vi "main.vi"() -> ()   [LabVIEW 2024]
uses:
  DataCluster.ctl
  <vilib>/userDefined/High Color/IMAQdx.ctl
  <vilib>/vision/Image Controls.llb/IMAQ Image.ctl
  DataQueue.ctl
  SensorCluster.ctl
  DataCluster_AC_PSU.ctl
  <vilib>/Platform/TimedLoop/XDataNode/timing_clust.ctl
  <vilib>/Platform/TimedLoop/XDataNode/nitl_modes.ctl
  <vilib>/Platform/TimedLoop/XDataNode/wakeup.ctl
  0b1114db-5621-4bc7-8375-4b786bff1f6f.vi
  4e5cdf46-f112-4ee0-b7be-49a859f3bfc5.vi
  2c923024-6a10-46aa-b2f6-1d0a339bce81.vi
  <extravilib>/ChannelInstances/Tag-t'DataCluster.ctl'/Read With Abort.vi
  <extravilib>/ChannelInstances/Tag-t'DataCluster.ctl'/Write With Abort.vi
  <extravilib>/ChannelInstances/Tag-t'DataCluster.ctl'/Instantiate.vi
  <extravilib>/ChannelInstances/Tag-t'DataCluster.ctl'/EndpointRead.vi
  <extravilib>/ChannelInstances/Stream-str/Instantiate.vi
  <vilib>/Platform/browser.llb/Open URL in Default Browser (string).vi
  <vilib>/Utility/file.llb/Write Delimited Spreadsheet (string).vi
  <extravilib>/ChannelInstances/Tag-t'DataCluster.ctl'/Endpoint.vi
  <vilib>/platform/TimedLoop/XDataNode/XDataNode.xnode
  <vilib>/vision/driver/NI_Vision_Acquisition_Software.lvlib
  <extravilib>/ChannelInstances/Tag-t'DataCluster.ctl'.lvlib
  <vilib>/Platform/TimedLoop/XDataNode/XDNodeRunTimeDep.lvlib
  <resource>/objmgr/imaqdx.rc
panel:
  out "Galium Control":string="Galium Control" caption="Version"
  in  "Save Snapshot":bool
  out "Overload":bool caption="System Overloaded!"
  out "error out 3":errorcluster
  out "Auto Tune PID gains":T1
  out "TuneComplete":bool caption="Done"
  in  "AutoTune":bool
  out "error out 2":errorcluster
  out "error out":errorcluster
  out "T_Log":string="00:30:00" caption="Sample Duration"
  out "version":string="version 0.0.0.1" caption="Version"
  in  "Start":bool
  out "Title":string="BioSIM" caption="Version"
  out "cDAQ_Time":u32(graph) caption="DAQ - Process Time"
  out "DP_Overhead":i64(graph)=499 caption="Data Acquisition - Overhead"
  in  "DataCluster":T2={"Core"={"Current VI Reference"=refnum, "Close Panel on Exit?"=FALSE, "Exit"=FALSE, "Initialized?"=FALSE}, "Connections"={"cDAQ DO"={"Task"="", "Connected"=FALSE, "Active"=FALSE, "ID"=""}, "cDAQ AO"={"Task"="", "Connected"=FALSE, "Active"=FALSE, "ID"=""}, "cDAQ AI"={"Task"="", "Connected"=FALSE, "Active"=FALSE, "ID"=""}, "Camera"={"Session"="", "Connected"=FALSE, "Active"=FALSE, "Placeholder"=refnum}, "Humidity"={"Port"="", "Connected"=FALSE, "Active"=FALSE}}, "Data Acquisition"={"Setup"={"Label"="", "Operator"="", "Notes"="", "CircTemp"=1.0, "FlowRate"=1.0}, "Camera"={"Image"=refnum, "Save Image"=refnum, "Image Frequency"=20, "Rectangle"={"Left"=0, "Top"=0, "Right"=0, "Bottom"=0, "Rotation"=0.0}, "Calibration"={"Top Left"={"X"=0.0, "Y"=0.0}, "Top Right"={"X"=0.0, "Y"=0.0}, "Bottom Left"={"X"=0.0, "Y"=0.0}, "Bottom Right"={"X"=0.0, "Y"=0.0}, "Fixpoint"={"X"=0.0, "Y"=0.0}, "Scan Area"=0.0, "Fixpoint Area"=0.0, "Well Pixels"=[], "Valid"=FALSE}, "FocusPos"=0, "Display Mapping"=10}, "Thermistor"={"Sample Size"=1, "Calibration"={"B0.100"=[], "R25"=[], "c"=[], "State"=[], "V_S"=5.0, "R_S"=100.0}, "Timing Mode"=14713}, "Partition"={"Data"=[], "Cell Label"="", "Cell Color"=0, "Height"=10, "Width"=16, "Grid"=[]}, "Queue"={"Queue"=refnum, "Size"=1}, "Sample Rate"=20, "Active"=FALSE, "Ready"=FALSE, "Graph Mode"=0, "Gradient Buffer"=2}, "Control"={"Sample Rate"=1, "LogStart ms"=0, "AC PSU"={"Voltage"=0.0, "Frequency"=0.0, "State"={"15+16 - Waveform"=0, "17 - Freq Control EN"=FALSE, "18 - Voltage Output"=FALSE, "19 - Output Mode"=0, "20 - Mode Control EN"=FALSE, "21 - AC Control EN"=FALSE, "24 - DC Control EN"=FALSE, "25 - DC Polarity Bias"=FALSE}}, "DC PSU"={"Voltage"=0.0, "Active"=FALSE, "Pulse Size"=0.0, "Pulse Duration"=0.0, "Voltage Set"=0.0}, "Computer Vision"={"Target Pos"=0.0, "Current Pos"=0.0, "Processing"=refnum, "Range"={"Lower value"=128.0, "Upper value"=255.0}, "MinArea"=2, "16-bit Conversion Method"=10, "Display Image"=10, "Binary"=refnum, "Gain"=0.0, "Exposure time"=0.0}, "PID"={"AutoPID"=FALSE, "Gains"={"proportional gain (Kc)"=1.0, "integral time (Ti, min)"=0.01, "derivative time (Td, min)"=0.0}, "autotuning parameters"={"controller type"=1, "relay cycles"=3, "relay amplitude"=1.0, "control specification"=2, "PV noise level"=0.1}, "Show Controls"=FALSE}}, "Manual Temp Control"={"TargetTemp"=1.0, "Mode"=0, "Active"=FALSE}} {"Manual Temp Control"."Mode" items=["Cool", "Heat"]; "Manual Temp Control"."TargetTemp" min=-40.0 max=40.0 step=0.5 format="%#_g °C"; "Control"."PID"."autotuning parameters"."PV noise level" format="%.2f"; "Control"."PID"."autotuning parameters"."control specification" items=["normal", "fast", "slow"]; "Control"."PID"."autotuning parameters"."relay amplitude" format="%.2f"; "Control"."PID"."autotuning parameters"."controller type" items=["PID", "PI", "P"]; "Control"."PID"."Gains"."derivative time (Td, min)" format="%.3f"; "Control"."PID"."Gains"."integral time (Ti, min)" format="%.3f"; "Control"."PID"."Gains"."proportional gain (Kc)" format="%.3f"; "Control"."Computer Vision"."Display Image" items=["Default", "Computer Vision"]; "Control"."Computer Vision"."16-bit Conversion Method" items=["Default"=10, "Most Significant Bits"=11, "Full Dynamic"=12, "Downshift"=13, "Given Range"=14, "90% Dynamic"=15, "Given Percent Range"=16]; "Control"."Computer Vision"."Range"."Upper value" format="%.2f"; "Control"."Computer Vision"."Range"."Lower value" format="%.2f"; "Control"."AC PSU"."State"."19 - Output Mode" items=["Constant Voltage", "Constant Current"]; "Control"."AC PSU"."State"."15+16 - Waveform" items=["Sine", "Square", "Triangle"]; "Control"."Sample Rate" min=1 max=20 step=1 format="%.0f Samples/sec"; "Data Acquisition"."Gradient Buffer" min=2 max=30 step=1; "Data Acquisition"."Graph Mode" items=["Thermistor Temperature", "Camera Temperature"]; "Data Acquisition"."Thermistor"."Timing Mode" items=["Automatic"=16097, "High Resolution"=10195, "High Speed"=14712, "Best 50 Hz Rejection"=14713, "Best 60 Hz Rejection"=14714, "Custom"=10137]; "Data Acquisition"."Thermistor"."Calibration"."R_S" min=0.1 max=1000.0 format="%#_g kOhm"; "Data Acquisition"."Thermistor"."Calibration"."V_S" min=5.0 max=48.0 format="%#_g V"; "Data Acquisition"."Thermistor"."Calibration"."R25" min=0.1 max=1000.0 format="%#_g kOhm"; "Data Acquisition"."Thermistor"."Calibration"."B0.100" min=100.0 max=10000.0 format="%#_g K"; "Data Acquisition"."Thermistor"."Sample Size" min=1 max=200; "Data Acquisition"."Sample Rate" min=20 max=240 format="%.0f samples/min"; "Data Acquisition"."Queue"."Size" min=1 max=200; "Data Acquisition"."Camera"."Display Mapping" items=["Default"=10, "Most Significant Bits"=11, "Full Dynamic"=12, "Downshift"=13, "Given Range"=14, "90% Dynamic"=15, "Given Percent Range"=16]; "Data Acquisition"."Camera"."Calibration"."Fixpoint"."Y" format="%.2f"; "Data Acquisition"."Camera"."Calibration"."Fixpoint"."X" format="%.2f"; "Data Acquisition"."Camera"."Calibration"."Top Left"."Y" format="%.2f"; "Data Acquisition"."Camera"."Calibration"."Top Left"."X" format="%.2f"; "Data Acquisition"."Camera"."Calibration"."Top Right"."Y" format="%.2f"; "Data Acquisition"."Camera"."Calibration"."Top Right"."X" format="%.2f"; "Data Acquisition"."Camera"."Calibration"."Bottom Left"."Y" format="%.2f"; "Data Acquisition"."Camera"."Calibration"."Bottom Left"."X" format="%.2f"; "Data Acquisition"."Camera"."Calibration"."Bottom Right"."Y" format="%.2f"; "Data Acquisition"."Camera"."Calibration"."Bottom Right"."X" format="%.2f"; "Data Acquisition"."Camera"."Rectangle"."Rotation" min=-90.0 max=90.0 step=1.0 format="%.2f"; "Data Acquisition"."Camera"."Rectangle"."Left" scale=0.0..1024.0; "Data Acquisition"."Camera"."Rectangle"."Right" scale=0.0..1024.0; "Data Acquisition"."Camera"."Image Frequency" min=1 max=60 step=1; "Data Acquisition"."Setup"."FlowRate" min=0.0 max=500.0 format="%#_g L/min"; "Data Acquisition"."Setup"."CircTemp" min=-40.0 max=40.0 step=0.5 format="%#_g °C"}
  in  "Help":bool
  out "DC Volt":dbl[unit](graph)
  out "Temps":dbl[unit](graph)
  out "Processing Feed":T4(plugin-control)
  out "Camera Feed":T4(plugin-control)
  out "Air Temp.":dbl format="%#_g °C"
  out "Dewpoint":dbl format="%#_g °C"
  out "Position":dbl caption="Average Position" format="%#.6f"
  out "Temp":dbl[unit]=273.15 caption="Temperature" format="%#.6f"
  out "Humidity Status":string
  out "Temp Status":string
  out "Humidity":dbl format="%#.6f %%"
  in  "Pulse":bool
  out "DC_Status":string
  in  "DC_Voltage_Slide":u32(slide) scale=0.0..100.0
  in  "DC_Voltage":dbl[unit] caption="DC Voltage" min=0.0 max=1500.0 format="%#.0f"
  out "AC_Status":string
  in  "AC_Voltage_Slide":u32(slide) scale=0.0..100.0
  in  "AC_Freq":dbl[unit]=100.0 caption="AC Frequency" min=100.0 max=10000.0 format="%#.0f"
  in  "AC_Voltage":dbl[unit] caption="AC Voltage" min=0.0 max=10000.0
  in  "AC_Freq_Slide":u32(slide) scale=0.0..100.0
  out "StatusString":string="Closing System"
  # "Bioaerosol Simulation Chamber"
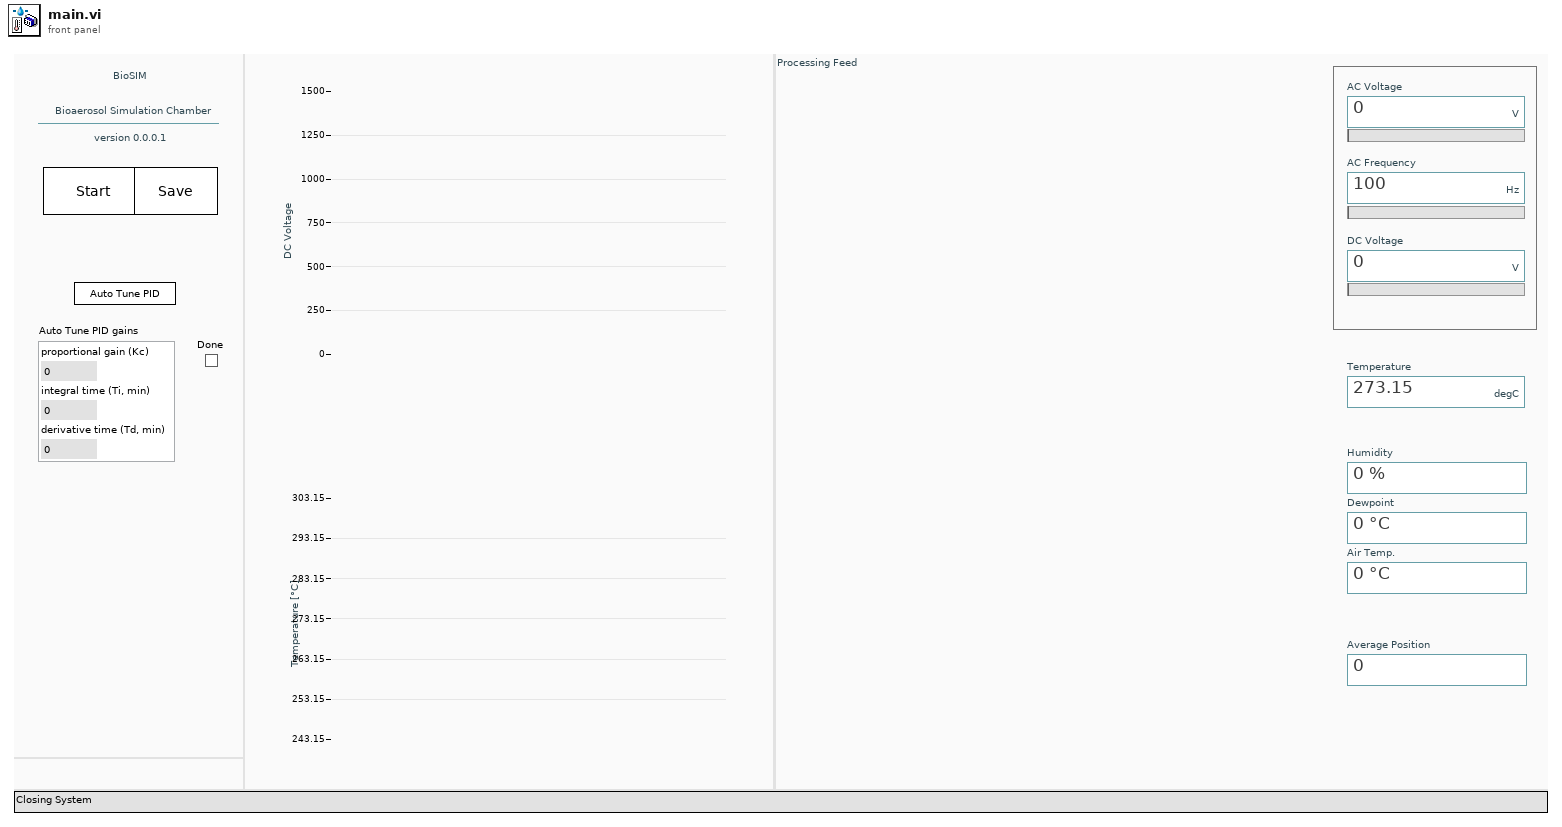
[diagram p1: front panel]
types:
  T1 = cluster{"proportional gain (Kc)":dbl, "integral time (Ti, min)":dbl, "derivative time (Td, min)":dbl}
  T2 = typedef "DataCluster.ctl" = cluster{"Core":cluster{"Current VI Reference":refnum<vi>, "Close Panel on Exit?":bool, "Exit":bool, "Initialized?":bool}, "Connections":cluster{"cDAQ DO":cluster{"Task":refnum<k21>, "Connected":bool, "Active":bool, "ID":string}, "cDAQ AO":cluster{"Task":refnum<k21>, "Connected":bool, "Active":bool, "ID":string}, "cDAQ AI":cluster{"Task":refnum<k21>, "Connected":bool, "Active":bool, "ID":string}, "Camera":cluster{"Session":T3, "Connected":bool, "Active":bool, "Placeholder":T4}, "Humidity":cluster{"Port":refnum<visa-resource-name>, "Connected":bool, "Active":bool}}, "Data Acquisition":cluster{"Setup":cluster{"Label":string, "Operator":string, "Notes":string, "CircTemp":dbl, "FlowRate":dbl}, "Camera":cluster{"Image":T4, "Save Image":T4, "Image Frequency":i32, "Rectangle":T5, "Calibration":cluster{"Top Left":T6, "Top Right":T6, "Bottom Left":T6, "Bottom Right":T6, "Fixpoint":T6, "Scan Area":dbl, "Fixpoint Area":dbl, "Well Pixels":cluster{"X":i32, "Y":i32}[][], "Valid":bool}, "FocusPos":u32, "Display Mapping":u32}, "Thermistor":cluster{"Sample Size":i32, "Calibration":cluster{"B0.100":dbl[], "R25":dbl[], "c":dbl[][], "State":bool[], "V_S":dbl, "R_S":dbl}, "Timing Mode":i32}, "Partition":cluster{"Data":string[][], "Cell Label":string, "Cell Color":u32, "Height":i32, "Width":i32, "Grid":string[][]}, "Queue":cluster{"Queue":refnum<queue>, "Size":i32}, "Sample Rate":i32, "Active":bool, "Ready":bool, "Graph Mode":u16, "Gradient Buffer":i32}, "Control":cluster{"Sample Rate":i32, "LogStart ms":u32, "AC PSU":cluster{"Voltage":dbl[unit], "Frequency":dbl[unit], "State":T7}, "DC PSU":cluster{"Voltage":dbl[unit], "Active":bool, "Pulse Size":dbl[unit], "Pulse Duration":dbl[unit], "Voltage Set":dbl[unit]}, "Computer Vision":cluster{"Target Pos":dbl, "Current Pos":dbl, "Processing":T4, "Range":cluster{"Lower value":sgl, "Upper value":sgl}, "MinArea":i32, "16-bit Conversion Method":u32, "Display Image":u32, "Binary":T4, "Gain":dbl, "Exposure time":dbl}, "PID":cluster{"AutoPID":bool, "Gains":cluster{"proportional gain (Kc)":dbl, "integral time (Ti, min)":dbl, "derivative time (Td, min)":dbl}, "autotuning parameters":cluster{"controller type":u16, "relay cycles":i32, "relay amplitude":dbl, "control specification":u16, "PV noise level":dbl}, "Show Controls":bool}}, "Manual Temp Control":cluster{"TargetTemp":dbl, "Mode":u16, "Active":bool}}
  T3 = typedef "IMAQdx.ctl" = refnum<k21>
  T4 = typedef "IMAQ Image.ctl" = refnum<image>
  T5 = typedef "IMAQ Rectangle" = cluster{"Left":i32, "Top":i32, "Right":i32, "Bottom":i32, "Rotation":dbl}
  T6 = typedef "IMAQ Point" = cluster{"X":sgl, "Y":sgl}
  T7 = typedef "DataCluster_AC_PSU.ctl" = cluster{"15+16 - Waveform":u16, "17 - Freq Control EN":bool, "18 - Voltage Output":bool, "19 - Output Mode":u16, "20 - Mode Control EN":bool, "21 - AC Control EN":bool, "24 - DC Control EN":bool, "25 - DC Polarity Bias":bool}
  T8 = enum32{"Invalid", "Standard", "Closed", "Hidden", "Minimized", "Maximized"}
  T9 = cluster{"Top Left":T6, "Top Right":T6, "Bottom Left":T6, "Bottom Right":T6, "Fixpoint":T6, "Scan Area":dbl, "Fixpoint Area":dbl, "Well Pixels":cluster{"X":i32, "Y":i32}[][], "Valid":bool}
  T10 = enum32{"invalid app kind", "Development System", "Run Time System", "Student Edition", "Embedded LabVIEW", "Evaluation", "Custom"}
  T11 = enum8{"Enabled", "Disabled", "Disabled and Grayed Out"}
  T12 = typedef "Stream-str.lvlib/)Channel.ctl" = refnum<queue>
  T13 = cluster{"Shift":bool, "Ctrl":bool, "Alt":bool, "Cmd":bool, "Opt":bool}
  T14 = typedef "Image Type" = u32
  T15 = enum16{"Faild to connect", "Connected", "Port wrong baud rate"}
  T16 = typedef "Tag-t'DataCluster.ctl'.lvlib/))Channel.ctl" = refnum<queue>
  T17 = typedef "XDNodeRunTimeDep.lvlib/timing_clust.ctl" = cluster{"Expected End [f-1]":u64, "Actual End [f-1]":u64, "Finished Late? [f-1]":bool, "Expected End [i-1]":u64, "Actual End [i-1]":u64, "Finished Late? [i-1]":bool, "Expected Start [i]":u64, "Actual Start [i]":u64, "Expected Start [f]":u64, "Actual Start [f]":u64, "Source Name":string, "Structure Name":string, "Period":i64, "Deadline":i64, "Offset":i64, "Start":i64, "Priority":i32, "Timeout":i32, "Mode":T18, "Wakeup Reason":T19, "Error":errorcluster, "Source Type":string, "Secondary Source Type":string, "Global End Time":u64, "Global Start Time":u64, "Frame Duration":u64, "Iteration Duration":u64, "Assigned CPU":i32, "I/O Scan Engine Mode":u32}
  T18 = typedef "XDNodeRunTimeDep.lvlib/nitl_modes.ctl" = enum32{"No Change", "Process missed periods, maintain original phase", "Discard missed periods, maintain original phase", "Process missed periods, ignore original phase", "Discard missed periods, ignore original phase"}
  T19 = typedef "XDNodeRunTimeDep.lvlib/wakeup.ctl" = enum32{"Normal", "Aborted", "Asynchronous wakeup", "Timing source error", "Timed loop error", "Timeout"}
  T20 = cluster{"tuning completed?":bool, "PID gains out":cluster{"proportional gain (Kc)":dbl, "integral time (Ti, min)":dbl, "derivative time (Td, min)":dbl}}
  T21 = typedef "SensorCluster.ctl" = cluster{"Temp":dbl[unit], "AC V":dbl[unit], "AC Freq":dbl[unit], "DC V":dbl[unit], "Temp Readings":dbl[], "Voltage Readings":dbl[], "CMH":cluster{"Humidity":dbl, "Dewpoint":dbl, "Air Temp":dbl}}
  T22 = cluster{"Humidity":dbl, "Dewpoint":dbl, "Air Temp":dbl}
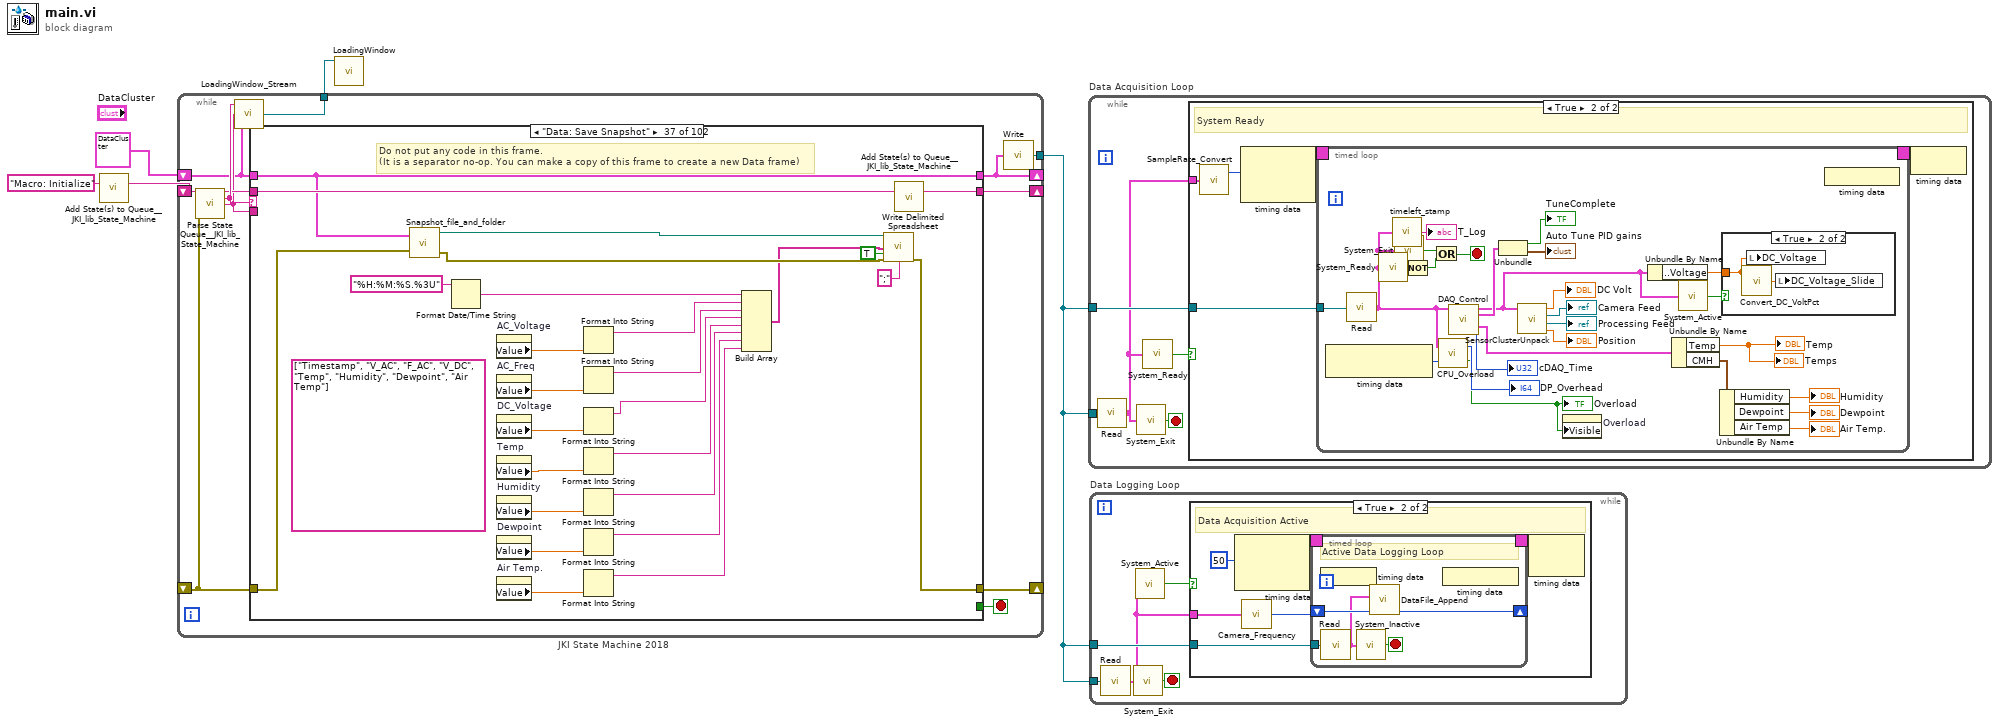
[diagram p0: block diagram]
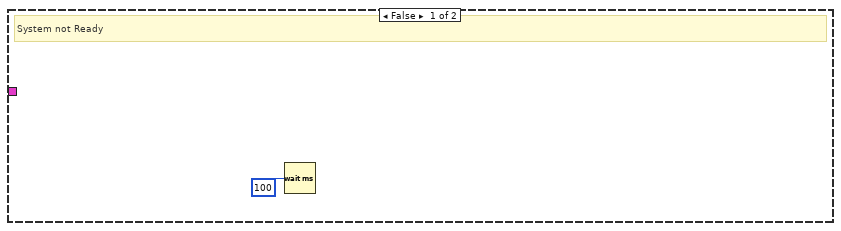
[diagram p2: hidden frame]
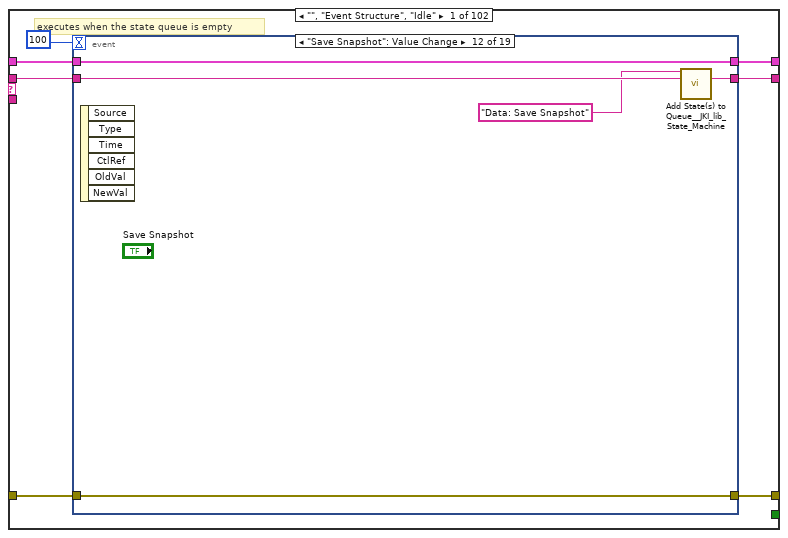
[diagram p4: hidden frame]
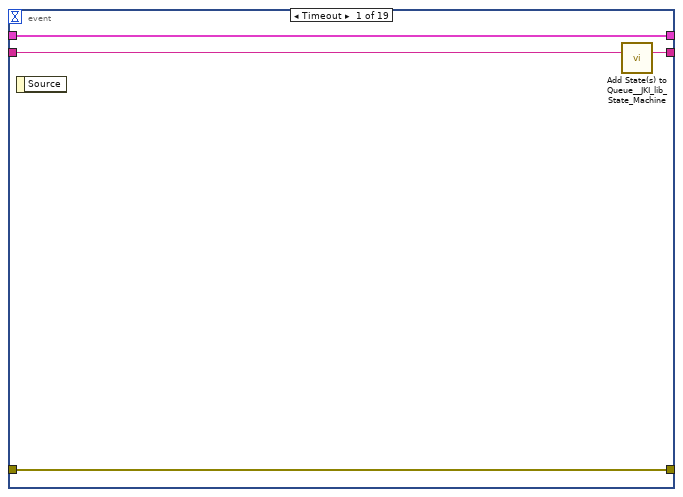
[diagram p5: hidden frame]
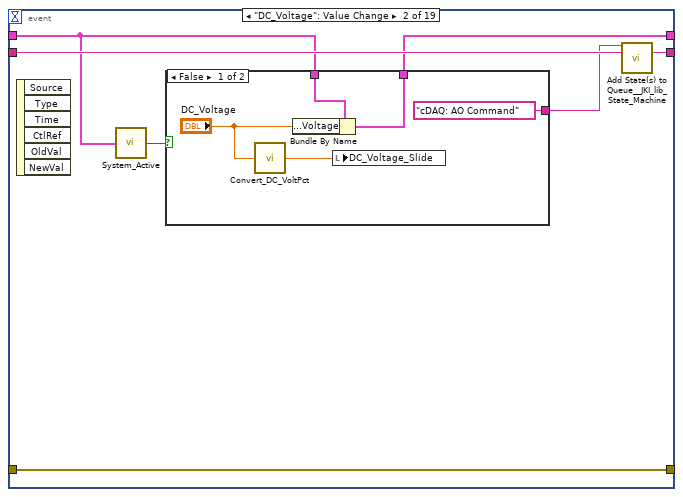
[diagram p6: hidden frame]
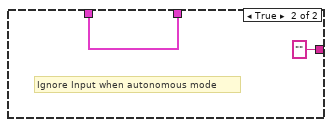
[diagram p7: hidden frame]
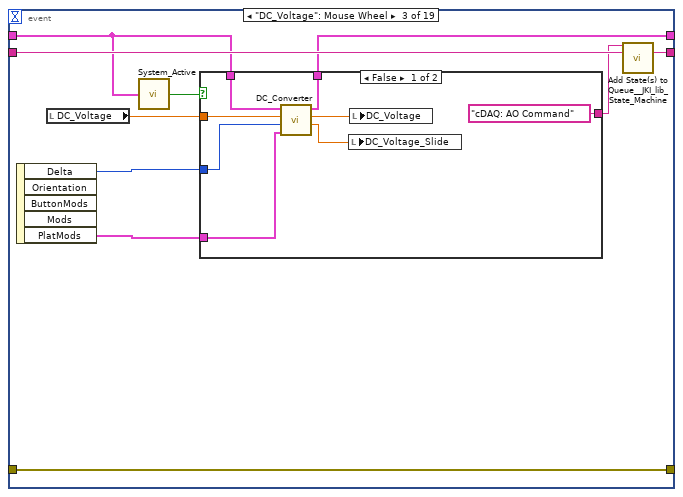
[diagram p8: hidden frame]
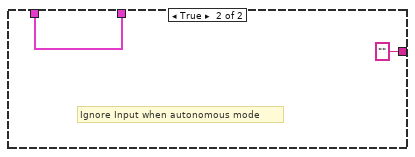
[diagram p9: hidden frame]
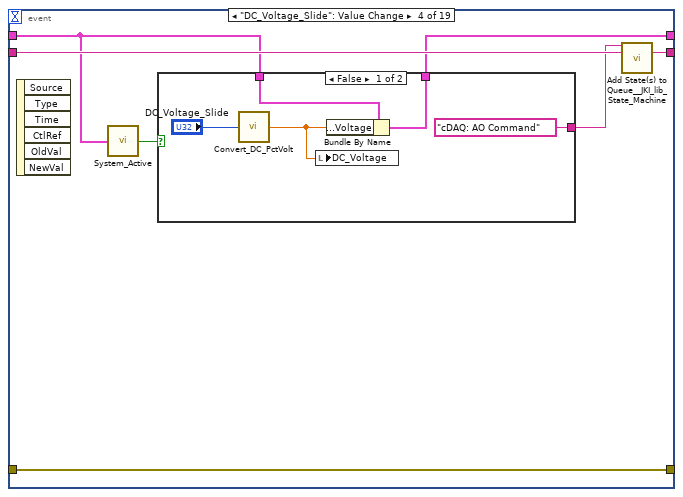
[diagram p10: hidden frame]
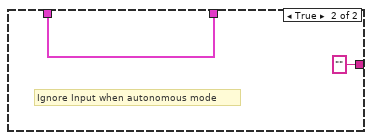
[diagram p11: hidden frame]
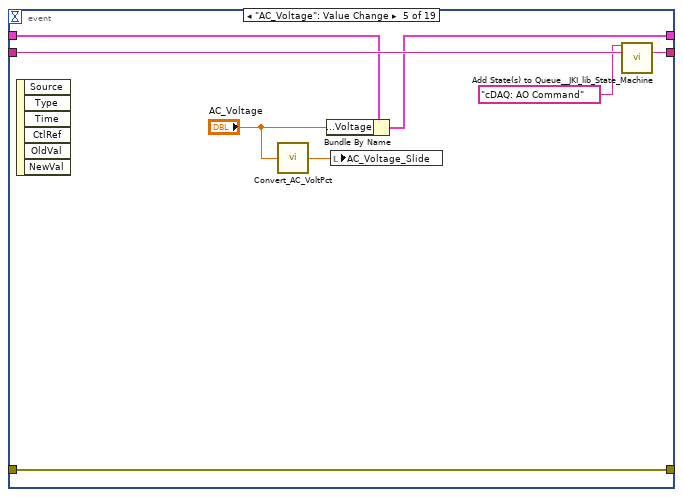
[diagram p12: hidden frame]
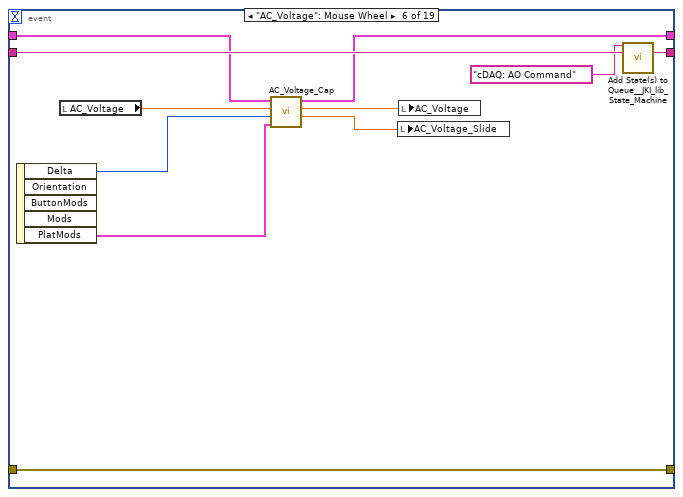
[diagram p13: hidden frame]
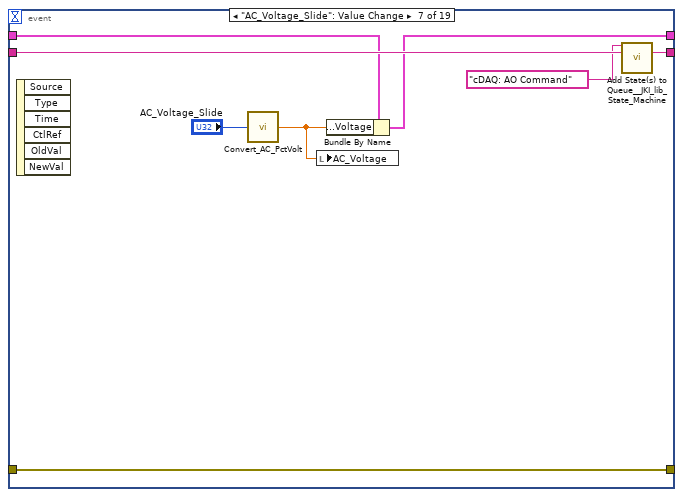
[diagram p14: hidden frame]
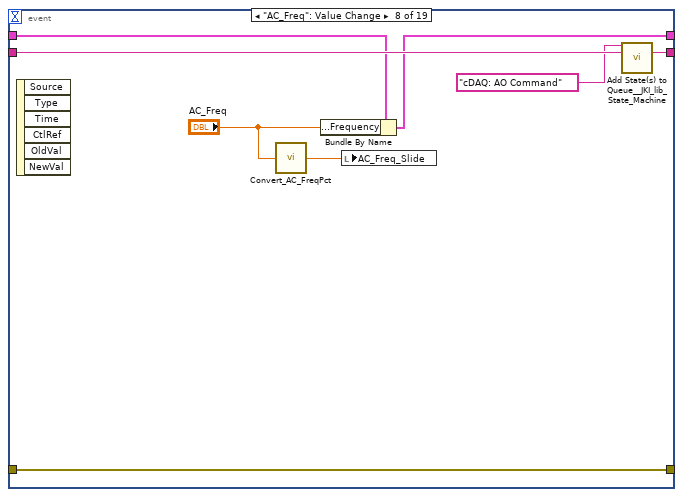
[diagram p15: hidden frame]
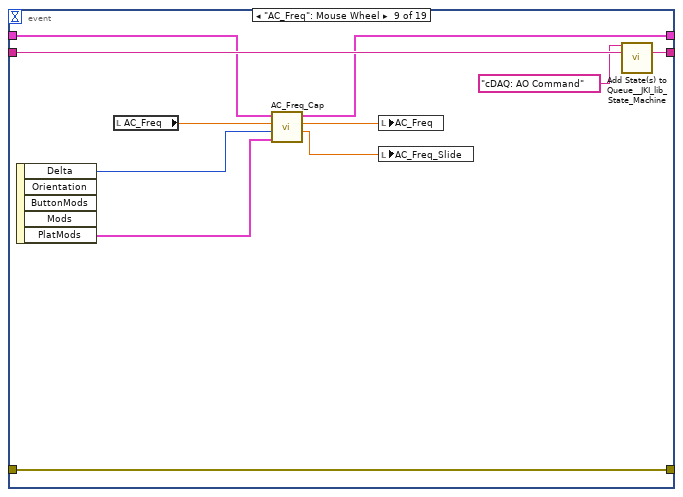
[diagram p16: hidden frame]
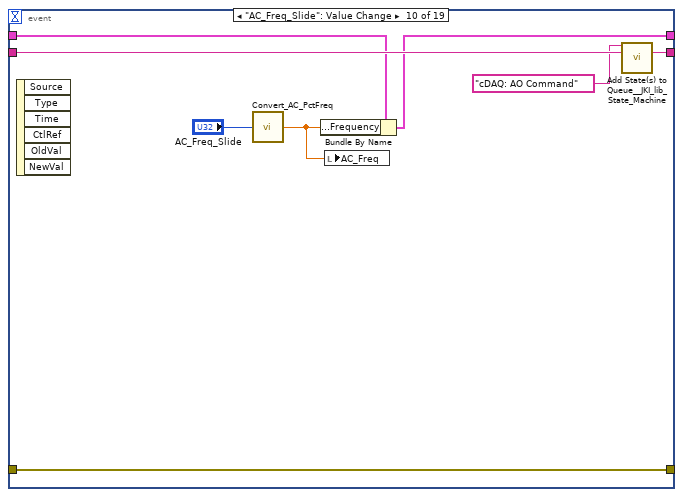
[diagram p17: hidden frame]
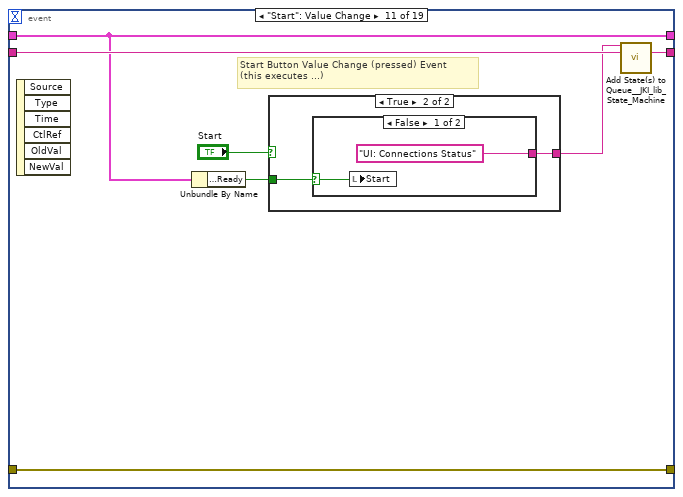
[diagram p18: hidden frame]
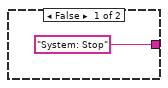
[diagram p19: hidden frame]
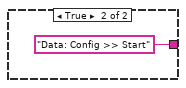
[diagram p20: hidden frame]
diagram:
  n1 = call <vilib>:"Add State(s) to Queue__JKI_lib_State_Machine.vi"("State(s) in (\"\")"="Macro: Initialize") -> ("States Out"=w5:string)  [unwired: 14 in]
  n2 = while "JKI State Machine 2018" {
    shift-right: [w10] -> _
    shift-left: T2 {"Core"={"Current VI Reference"=refnum, "Close Panel on Exit?"=FALSE, "Exit"=FALSE, "Initialized?"=FALSE}, "Connections"={"cDAQ DO"={"Task"="", "Connected"=FALSE, "Active"=FALSE, "ID"=""}, "cDAQ AO"={"Task"="", "Connected"=FALSE, "Active"=FALSE, "ID"=""}, "cDAQ AI"={"Task"="", "Connected"=FALSE, "Active"=FALSE, "ID"=""}, "Camera"={"Session"="", "Connected"=FALSE, "Active"=FALSE, "Placeholder"=refnum}, "Humidity"={"Port"="", "Connected"=FALSE, "Active"=FALSE}}, "Data Acquisition"={"Setup"={"Label"="", "Operator"="", "Notes"="", "CircTemp"=0.0, "FlowRate"=0.0}, "Camera"={"Image"=refnum, "Save Image"=refnum, "Image Frequency"=0, "Rectangle"={"Left"=0, "Top"=0, "Right"=0, "Bottom"=0, "Rotation"=0.0}, "Calibration"={"Top Left"={"X"=0.0, "Y"=0.0}, "Top Right"={"X"=0.0, "Y"=0.0}, "Bottom Left"={"X"=0.0, "Y"=0.0}, "Bottom Right"={"X"=0.0, "Y"=0.0}, "Fixpoint"={"X"=0.0, "Y"=0.0}, "Scan Area"=0.0, "Fixpoint Area"=0.0, "Well Pixels"=[], "Valid"=FALSE}, "FocusPos"=0, "Display Mapping"=0}, "Thermistor"={"Sample Size"=0, "Calibration"={"B0.100"=[], "R25"=[], "c"=[], "State"=[], "V_S"=0.0, "R_S"=0.0}, "Timing Mode"=0}, "Partition"={"Data"=[], "Cell Label"="", "Cell Color"=0, "Height"=0, "Width"=0, "Grid"=[]}, "Queue"={"Queue"=refnum, "Size"=0}, "Sample Rate"=0, "Active"=FALSE, "Ready"=FALSE, "Graph Mode"=0, "Gradient Buffer"=0}, "Control"={"Sample Rate"=0, "LogStart ms"=0, "AC PSU"={"Voltage"=0.0, "Frequency"=0.0, "State"={"15+16 - Waveform"=0, "17 - Freq Control EN"=FALSE, "18 - Voltage Output"=FALSE, "19 - Output Mode"=0, "20 - Mode Control EN"=FALSE, "21 - AC Control EN"=FALSE, "24 - DC Control EN"=FALSE, "25 - DC Polarity Bias"=FALSE}}, "DC PSU"={"Voltage"=0.0, "Active"=FALSE, "Pulse Size"=0.0, "Pulse Duration"=0.0, "Voltage Set"=0.0}, "Computer Vision"={"Target Pos"=0.0, "Current Pos"=0.0, "Processing"=refnum, "Range"={"Lower value"=128.0, "Upper value"=255.0}, "MinArea"=2, "16-bit Conversion Method"=10, "Display Image"=10, "Binary"=refnum, "Gain"=0.0, "Exposure time"=0.0}, "PID"={"AutoPID"=FALSE, "Gains"={"proportional gain (Kc)"=0.0, "integral time (Ti, min)"=0.0, "derivative time (Td, min)"=0.0}, "autotuning parameters"={"controller type"=1, "relay cycles"=3, "relay amplitude"=1.0, "control specification"=2, "PV noise level"=0.1}, "Show Controls"=FALSE}}, "Manual Temp Control"={"TargetTemp"=0.0, "Mode"=0, "Active"=FALSE}} ("DataCluster") -> [w7]
    shift-right: [w14] -> _
    shift-left: _ -> [w12]
    shift-right: [w6] -> _
    shift-left: w5 -> [w15]
    tunnel: [w11] -> w1
    tunnel: [w9] -> w2
    stop <- w13 stop-if-true
    n3 = call <vilib>:"Parse State Queue__JKI_lib_State_Machine.vi"("State Queue"=w15, "Error In (no error)"=w12) -> ("Remaining States"=w16:string, "Current State"=w17:string, "Arguments"=w8:string)  [unwired: 11 in]
    n4 = call "LoadingWindow_Stream.vi"("DataCluster"=w7, "Arguments"=w8, "Current State"=w17) -> ("Channel out"=w9:T12)
    n5 = case shown="\"Data: Save Snapshot\"" w17 {
      selector: w17 -> [_ _ w257 _ _ _ _ _ _ _ _ _ _ _ _ _ _ _ _ _ _ _ _ _ _ _ _ _ _ _ _ _ _ _ _ _ _ _ _ _ _ _ _ _ _ _ _ _ _ _ _ _ _ _ _ _ _ _ _ _ _ _ _ _ _ _ _ _ _ _ _ _ _ _ _ _ _ _ _ _ _ _ _ _ _ _ _ _ _ _ _ _ _ _ _ _ _ _ _ _ _ _]
      tunnel: w16 -> [w24 w256 w261 w275 w289 w296 w303 w307 w316 w329 w333 w342 w357 w364 w374 w380 w385 w389 w397 w406 w419 w436 w444 w457 w468 w474 w480 w486 w493 w498 w504 w509 w528 w534 w549 w564 w594 w598 w603 w612 w622 w634 w639 w645 w650 w655 w660 w667 w675 w683 w687 w691 w699 w712 w721 w736 w743 w750 w766 w789 w804 w812 w834 w838 w849 w866 w873 w877 w892 w897 w911 w917 w923 w935 w956 w963 w971 w977 w988 w1009 w1026 w1042 w1049 w1060 w1065 w1072 w1079 w1094 w1114 w1125 w1194 w1199 w1203 w1214 w1225 w1229 w1235 w1242 w1246 w1250 w1254 w1258]
      tunnel: w8 -> [_ _ _ w271 w283 _ _ _ _ _ _ _ w353 w358 _ w376 _ _ _ _ _ _ w439 w452 _ _ _ _ _ _ _ _ _ _ _ _ _ _ _ _ _ _ _ _ _ _ _ w664 _ _ _ _ _ _ _ _ _ _ _ _ _ _ _ _ _ _ _ _ _ w893 _ _ w919 w931 _ w959 _ w972 w984 w1005 w1022 _ w1045 w1056 w1061 _ w1075 w1090 w1109 w1119 _ _ _ _ _ _ _ _ _ _ _ _]
      tunnel: w7 -> [w22 w253 w259 w273 w287 w293 w299 w304 w313 w318 w330 w334 w352 w361 w371 w377 w381 w386 w390 w403 w412 w424 w441 w454 w466 w472 w478 w483 w491 w494 w502 w507 w514 w530 w543 w553 w592 w595 w600 w609 w616 w631 w636 w642 w647 w652 w657 w663 w670 w680 w684 w688 w697 w710 w714 w733 w740 w745 w762 w785 w802 w806 w832 w835 w840 w864 w867 w874 w886 w895 w909 w915 w920 w932 w953 w961 w968 w974 w985 w1006 w1023 w1039 w1047 w1058 w1063 w1068 w1077 w1092 w1112 w1121 w1191 w1197 w1201 w1212 w1222 w1226 w1232 w1239 w1243 w1247 w1251 w1255]
      tunnel: [w21 w254 w263 w268 w285 errorcluster {"status"=FALSE, "code"=0, "source"=""} ("error out") w301 w305 w314 w327 w331 w340 w355 w362 w372 w378 w383 w387 w392 w402 w416 w420 w442 w455 w463 w469 w476 w484 w488 w495 w500 w505 w512 w532 w536 w551 w586 w596 w601 w610 w620 w632 w637 w640 w648 w653 w658 w665 w673 w681 w685 w689 w694 w708 w716 w734 w738 w746 w758 w782 w799 w807 w830 w836 w842 w862 w869 w875 w890 w894 w908 w914 w921 w933 w954 w960 w969 w975 w986 w1007 w1024 w1040 w1046 w1057 w1062 w1070 w1076 w1091 w1110 w1122 w1192 w1195 w1200 w1211 w1223 w1227 w1233 w1240 w1244 w1248 w1252 w1256] -> w14
      tunnel: w12 -> [w20 w254 w262 w268 w285 w292 w301 w305 w314 w327 w331 w340 w355 w362 w372 w378 w383 w387 w394 w399 w416 w422 w442 w455 w463 w469 w476 w484 w489 w496 w501 w506 w510 w531 w537 w552 w591 w596 w601 w610 w620 w632 w637 w640 w648 w653 w658 w665 w673 w681 w685 w689 w695 w709 w717 w734 w741 w747 w763 w783 w800 w808 w831 w836 w842 w863 w870 w875 w890 w894 w908 w914 w921 w933 w954 w960 w969 w975 w986 w1007 w1024 w1040 w1046 w1057 w1062 w1070 w1076 w1091 w1111 w1123 w1192 w1196 w1200 w1211 w1223 w1227 w1233 w1240 w1244 w1248 w1252 w1256]
      tunnel: [w23 w255 w260 w274 w288 w295 w302 w306 w315 w328 w332 w341 w356 w363 w373 w379 w384 w388 w396 w405 w418 w435 w443 w456 w467 w473 w479 w485 w492 w497 w503 w508 w527 w533 w548 w563 w593 w597 w602 w611 w621 w633 w638 w644 w649 w654 w659 w666 w674 w682 w686 w690 w698 w711 w720 w735 w742 w749 w765 w788 w803 w811 w833 w837 w848 w865 w872 w876 w891 w896 w910 w916 w922 w934 w955 w962 w970 w976 w987 w1008 w1025 w1041 w1048 w1059 w1064 w1071 w1078 w1093 w1113 w1124 w1193 w1198 w1202 w1213 w1224 w1228 w1234 w1241 w1245 w1249 w1253 w1257] -> w6
      tunnel: [_ _ _ _ _ _ TRUE _ _ _ _ _ _ _ _ _ _ _ _ _ _ _ _ _ _ _ _ _ _ _ _ _ _ _ _ _ _ _ _ _ _ _ _ _ _ _ _ _ _ _ _ _ _ _ _ _ _ _ _ _ _ _ _ _ _ _ _ _ _ _ _ _ _ _ _ _ _ _ _ _ _ _ _ _ _ _ _ _ _ _ _ _ _ _ _ _ _ _ _ _ _ _] -> w13
      tunnel: [w19 w253 w259 w273 w287 w293 w297 w304 w313 w317 w330 w334 w351 w359 w368 w377 w381 w386 w395 w403 w417 w434 w440 w453 w465 w471 w477 w482 w490 w494 w499 w507 w514 w529 w543 w553 w592 w595 w600 w605 w615 w631 w635 w643 w646 w651 w656 w661 w668 w679 w684 w688 w696 w707 w713 w733 w739 w748 w761 w784 w801 w805 w829 w835 w844 w861 w867 w874 w886 w895 w909 w915 w920 w932 w953 w961 w968 w974 w985 w1006 w1023 w1039 w1047 w1058 w1063 w1068 w1077 w1092 w1112 w1121 w1191 w1197 w1201 w1212 w1222 w1226 w1231 w1238 w1243 w1247 w1251 w1255] -> w10
      frame "", "Event Structure", "Idle" {
        # "executes when the state queue is empty"
        n6 = event shown="[11] \"Save Snapshot\": Value Change" {
          selector: _ -> [_ _ _ _ _ _ _ _ _ _ _ _ _ _ _ _ _ _ _]
          dyn-events: _ -> [_ _ _ _ _ _ _ _ _ _ _ _ _ _ _ _ _ _ _]
          timeout: 100 ("Timeout") -> [_ _ _ _ _ _ _ _ _ _ _ _ _ _ _ _ _ _ _]
          tunnel: w24 -> [w28 w35 w52 w69 w84 w95 w103 w111 w122 w130 w137 w146 w155 w166 w171 w178 w189 w196 w252]
          tunnel: [w27 w34 w51 w68 w83 w94 w102 w110 w121 w129 w136 w145 w154 w165 w170 w177 w188 w195 w251] -> w23
          tunnel: w22 -> [w25 w30 w44 w64 w81 w92 w100 w108 w119 w127 w132 w148 w150 w163 w168 w173 w186 w191 w249]
          tunnel: [w26 w33 w50 w67 w82 w93 w101 w109 w120 w128 w135 w147 w153 w164 w169 w176 w187 w194 w250] -> w21
          tunnel: w20 -> [w26 w33 w50 w67 w82 w93 w101 w109 w120 w128 w135 w147 w153 w164 w169 w176 w187 w194 w250]
          tunnel: [w25 w32 w49 w66 w80 w91 w99 w107 w118 w126 w132 w148 w149 w163 w168 w175 w185 w190 w246] -> w19
          event Timeout {
            n7 = event-data() -> ()  [unwired: 1 in, 1 out]
            n8 = call <vilib>:"Add State(s) to Queue__JKI_lib_State_Machine.vi"("State(s) in (\"\")"=w28) -> ("States Out"=w27:string)  [unwired: 14 in]
          }
          event "DC_Voltage": Value Change {
            n9 = event-data() -> ()  [unwired: 1 in, 6 out]
            n10 = call "System_Active.vi"("DataCluster"=w30) -> ("Data Acquisition Active"=w29:bool)
            n11 = case shown="False" w29 {
              tunnel: w30 -> [w40 w42]
              tunnel: [w39 w42] -> w32
              tunnel: ["cDAQ: AO Command" ("State(s) in Front (\"\")") "" ("State(s) in Front (\"\")")] -> w31
              frame False {
                n12 = call "Convert_DC_VoltPct.vi"("DC_Volt"="DC_Voltage") -> ("DC_Volt%"=w38:dbl)
                n13 = Bundle By Name(cluster=w40, "Control.DC PSU.Voltage"="DC_Voltage") -> (w39:T2)
                n14 = local write "DC_Voltage_Slide"(w38) -> ()
              }
              frame True {
                # "Ignore Input when autonomous mode"
              }
            }
            n15 = call <vilib>:"Add State(s) to Queue__JKI_lib_State_Machine.vi"("State(s) in Front (\"\")"=w31, "State(s) in (\"\")"=w35) -> ("States Out"=w34:string)  [unwired: 13 in]
          }
          event "DC_Voltage": Mouse Wheel {
            n16 = event-data() -> ("Delta"=w48:i32, "PlatMods"=w45:T13)  [unwired: 1 in, 3 out]
            n17 = local read "DC_Voltage"() -> (w47:dbl[unit])
            n18 = call "System_Active.vi"("DataCluster"=w44) -> ("Data Acquisition Active"=w43:bool)
            n19 = case shown="False" w43 {
              tunnel: [w60 w62] -> w49
              tunnel: w48 -> [w58 _]
              tunnel: w47 -> [w57 _]
              tunnel: ["cDAQ: AO Command" ("State(s) in Front (\"\")") "" ("State(s) in Front (\"\")")] -> w46
              tunnel: w45 -> [w54 _]
              tunnel: w44 -> [w53 w62]
              frame False {
                n20 = call "DC_Converter.vi"("PlatMods"=w54, "Delta"=w58, "DC_Voltage"=w57, "DataCluster in"=w53) -> ("DC_Volt%"=w59:dbl, "Coerced Volt"=w56:dbl[unit], "DataCluster out"=w60:T2)  [unwired: 5 in]
                n21 = local write "DC_Voltage_Slide"(w59) -> ()
                n22 = local write "DC_Voltage"(w56) -> ()
              }
              frame True {
                # "Ignore Input when autonomous mode"
              }
            }
            n23 = call <vilib>:"Add State(s) to Queue__JKI_lib_State_Machine.vi"("State(s) in Front (\"\")"=w46, "State(s) in (\"\")"=w52) -> ("States Out"=w51:string)  [unwired: 13 in]
          }
          event "DC_Voltage_Slide": Value Change {
            n24 = event-data() -> ()  [unwired: 1 in, 6 out]
            n25 = call "System_Active.vi"("DataCluster"=w64) -> ("Data Acquisition Active"=w63:bool)
            n26 = case shown="False" w63 {
              tunnel: [w74 w76] -> w66
              tunnel: ["cDAQ: AO Command" ("State(s) in Front (\"\")") "" ("State(s) in Front (\"\")")] -> w65
              tunnel: w64 -> [w70 w76]
              frame False {
                n27 = call "Convert_DC_PctVolt.vi"("DC_Volt%"="DC_Voltage_Slide") -> ("DC_Volt"=w72:dbl[unit])
                n28 = local write "DC_Voltage"(w72) -> ()
                n29 = Bundle By Name(cluster=w70, "Control.DC PSU.Voltage"=w72) -> (w74:T2)
              }
              frame True {
                # "Ignore Input when autonomous mode"
              }
            }
            n30 = call <vilib>:"Add State(s) to Queue__JKI_lib_State_Machine.vi"("State(s) in Front (\"\")"=w65, "State(s) in (\"\")"=w69) -> ("States Out"=w68:string)  [unwired: 13 in]
          }
          event "AC_Voltage": Value Change {
            n31 = event-data() -> ()  [unwired: 1 in, 6 out]
            n32 = call "Convert_AC_VoltPct.vi"("AC_Volt"="AC_Voltage") -> ("AC_Volt%"=w78:dbl)
            n33 = Bundle By Name(cluster=w81, "Control.AC PSU.Voltage"="AC_Voltage") -> (w80:T2)
            n34 = local write "AC_Voltage_Slide"(w78) -> ()
            n35 = call <vilib>:"Add State(s) to Queue__JKI_lib_State_Machine.vi"("State(s) in Front (\"\")"="cDAQ: AO Command" ("State(s) in Front (\"\")"), "State(s) in (\"\")"=w84) -> ("States Out"=w83:string)  [unwired: 13 in]
          }
          event "AC_Voltage": Mouse Wheel {
            n36 = event-data() -> ("Delta"=w89:i32, "PlatMods"=w85:T13)  [unwired: 1 in, 3 out]
            n37 = local read "AC_Voltage"() -> (w88:dbl[unit])
            n38 = call "AC_Voltage_Cap.vi"("PlatMods"=w85, "Delta"=w89, "AC_Voltage"=w88, "DataCluster in"=w92) -> ("AC_Volt%"=w90:dbl, "lower limit"=w87:dbl[unit], "DataCluster out"=w91:T2)  [unwired: 5 in]
            n39 = local write "AC_Voltage_Slide"(w90) -> ()
            n40 = local write "AC_Voltage"(w87) -> ()
            n41 = call <vilib>:"Add State(s) to Queue__JKI_lib_State_Machine.vi"("State(s) in Front (\"\")"="cDAQ: AO Command" ("State(s) in Front (\"\")"), "State(s) in (\"\")"=w95) -> ("States Out"=w94:string)  [unwired: 13 in]
          }
          event "AC_Voltage_Slide": Value Change {
            n42 = event-data() -> ()  [unwired: 1 in, 6 out]
            n43 = call "Convert_AC_PctVolt.vi"("AC_Volt%"="AC_Voltage_Slide") -> ("AC_Volt"=w97:dbl[unit])
            n44 = local write "AC_Voltage"(w97) -> ()
            n45 = Bundle By Name(cluster=w100, "Control.AC PSU.Voltage"=w97) -> (w99:T2)
            n46 = call <vilib>:"Add State(s) to Queue__JKI_lib_State_Machine.vi"("State(s) in Front (\"\")"="cDAQ: AO Command" ("State(s) in Front (\"\")"), "State(s) in (\"\")"=w103) -> ("States Out"=w102:string)  [unwired: 13 in]
          }
          event "AC_Freq": Value Change {
            n47 = event-data() -> ()  [unwired: 1 in, 6 out]
            n48 = call "Convert_AC_FreqPct.vi"("Freq_Hz"="AC_Freq") -> ("Freq%"=w105:dbl)
            n49 = Bundle By Name(cluster=w108, "Control.AC PSU.Frequency"="AC_Freq") -> (w107:T2)
            n50 = local write "AC_Freq_Slide"(w105) -> ()
            n51 = call <vilib>:"Add State(s) to Queue__JKI_lib_State_Machine.vi"("State(s) in Front (\"\")"="cDAQ: AO Command" ("State(s) in Front (\"\")"), "State(s) in (\"\")"=w111) -> ("States Out"=w110:string)  [unwired: 13 in]
          }
          event "AC_Freq": Mouse Wheel {
            n52 = event-data() -> ("Delta"=w116:i32, "PlatMods"=w112:T13)  [unwired: 1 in, 3 out]
            n53 = local read "AC_Freq"() -> (w115:dbl[unit])
            n54 = call "AC_Freq_Cap.vi"("PlatMods"=w112, "Delta"=w116, "AC_Freq"=w115, "DataCluster in"=w119) -> ("Freq%"=w117:dbl, "lower limit"=w114:dbl[unit], "DataCluster out"=w118:T2)  [unwired: 5 in]
            n55 = local write "AC_Freq"(w114) -> ()
            n56 = local write "AC_Freq_Slide"(w117) -> ()
            n57 = call <vilib>:"Add State(s) to Queue__JKI_lib_State_Machine.vi"("State(s) in Front (\"\")"="cDAQ: AO Command" ("State(s) in Front (\"\")"), "State(s) in (\"\")"=w122) -> ("States Out"=w121:string)  [unwired: 13 in]
          }
          event "AC_Freq_Slide": Value Change {
            n58 = event-data() -> ()  [unwired: 1 in, 6 out]
            n59 = call "Convert_AC_PctFreq.vi"("Freq%"="AC_Freq_Slide") -> ("Freq_Hz"=w124:dbl[unit])
            n60 = Bundle By Name(cluster=w127, "Control.AC PSU.Frequency"=w124) -> (w126:T2)
            n61 = local write "AC_Freq"(w124) -> ()
            n62 = call <vilib>:"Add State(s) to Queue__JKI_lib_State_Machine.vi"("State(s) in Front (\"\")"="cDAQ: AO Command" ("State(s) in Front (\"\")"), "State(s) in (\"\")"=w130) -> ("States Out"=w129:string)  [unwired: 13 in]
          }
          event "Start": Value Change {
            # "Start Button Value Change (pressed) Event\n(this executes ...)"
            n63 = event-data() -> ()  [unwired: 1 in, 6 out]
            n64 = Unbundle By Name(w132) -> ("Data Acquisition.Ready"=w131:bool)
            n65 = case shown="True" "Start" {
              tunnel: ["System: Stop" ("State(s) in Front (\"\")") w140] -> w133
              tunnel: w131 -> [_ w139]
              frame False {
              }
              frame True {
                n66 = case shown="False" w139 {
                  selector: w139 -> [w141 _]
                  tunnel: ["UI: Connections Status" ("State(s) in Front (\"\")") "Data: Config >> Start" ("State(s) in Front (\"\")")] -> w140
                  frame False {
                    n67 = local write "Start"(w141) -> ()
                  }
                  frame True {
                  }
                }
              }
            }
            n68 = call <vilib>:"Add State(s) to Queue__JKI_lib_State_Machine.vi"("State(s) in Front (\"\")"=w133, "State(s) in (\"\")"=w137) -> ("States Out"=w136:string)  [unwired: 13 in]
          }
          event "Save Snapshot": Value Change {
            n69 = event-data() -> ()  [unwired: 1 in, 6 out]
            n70 = call <vilib>:"Add State(s) to Queue__JKI_lib_State_Machine.vi"("State(s) in Front (\"\")"="Data: Save Snapshot" ("State(s) in Front (\"\")"), "State(s) in (\"\")"=w146) -> ("States Out"=w145:string)  [unwired: 13 in]
          }
          event "AutoTune": Value Change {
            # "Start Button Value Change (pressed) Event\n(this executes ...)"
            n71 = event-data() -> ()  [unwired: 1 in, 6 out]
            n72 = Unbundle By Name(w150) -> ("Data Acquisition.Ready"=w151:bool)
            n73 = local write "Start"(w151) -> ()
            n74 = case shown="True" w151 {
              tunnel: ["UI: Connections Status" ("State(s) in Front (\"\")") "System: Start\nUI: Autotune >> Diable\nSystem: Disable Autotune" ("State(s) in Front (\"\")")] -> w152
              tunnel: w150 -> [w156 w160]
              tunnel: [w156 w159] -> w149
              frame False {
              }
              frame True {
                n75 = Bundle By Name(cluster=w160, "Control.PID.AutoPID"=TRUE) -> (w159:T2)
              }
            }
            n76 = call <vilib>:"Add State(s) to Queue__JKI_lib_State_Machine.vi"("State(s) in Front (\"\")"=w152, "State(s) in (\"\")"=w155) -> ("States Out"=w154:string)  [unwired: 13 in]
          }
          event "Help": Value Change {
            # "Exit Button Value Change (pressed) Event\n(this executes Macro: Exit to terminate the VI)"
            n77 = event-data() -> ()  [unwired: 1 in, 6 out]
            n78 = call <vilib>:"Add State(s) to Queue__JKI_lib_State_Machine.vi"("State(s) in Front (\"\")"="UI: Help >> About" ("State(s) in Front (\"\")"), "State(s) in (\"\")"=w166) -> ("States Out"=w165:string)  [unwired: 13 in]
          }
          event "Pulse": Value Change {
            # "DC Pulse Value Change (pressed) Event\n(this executes DC Pulse)"
            n79 = event-data() -> ()  [unwired: 1 in, 6 out]
            n80 = call <vilib>:"Add State(s) to Queue__JKI_lib_State_Machine.vi"("State(s) in Front (\"\")"="cDAQ: AO Pulse" ("State(s) in Front (\"\")"), "State(s) in (\"\")"=w171) -> ("States Out"=w170:string)  [unwired: 13 in]
          }
          event "DC_Status": Mouse Up {
            # "DC Status (pressed) Event\n(this toggles DC Output command)"
            n81 = event-data() -> ()  [unwired: 1 in, 8 out]
            n82 = call "System_Active.vi"("DataCluster"=w173) -> ("Data Acquisition Active"=w172:bool)
            n83 = case shown="False" w172 {
              tunnel: w173 -> [w181 w183]
              tunnel: [w180 w183] -> w175
              tunnel: [w179 "" ("State out")] -> w174
              frame False {
                n84 = call "DC_Toggle.vi"("DataCluster in"=w181) -> ("State out"=w179:string, "DataCluster out"=w180:T2)  [unwired: 9 in]
              }
              frame True {
              }
            }
            n85 = call <vilib>:"Add State(s) to Queue__JKI_lib_State_Machine.vi"("State(s) in Front (\"\")"=w174, "State(s) in (\"\")"=w178) -> ("States Out"=w177:string)  [unwired: 13 in]
          }
          event "AC_Status": Mouse Up {
            # "AC Status (pressed) Event\n(This toggles the AC PSU output)"
            n86 = event-data() -> ()  [unwired: 1 in, 8 out]
            n87 = call "AC_Toggle.vi"("DataCluster in"=w186) -> ("State out"=w184:string, "DataCluster out"=w185:T2)  [unwired: 9 in]
            n88 = call <vilib>:"Add State(s) to Queue__JKI_lib_State_Machine.vi"("State(s) in Front (\"\")"=w184, "State(s) in (\"\")"=w189) -> ("States Out"=w188:string)  [unwired: 13 in]
          }
          event Menu Selection (User) {
            # "Shortcut Menu (pressed) Event\n(this executes events, based on selected menu item)"
            n89 = event-data() -> ("ItemTag"=w193:string)  [unwired: 1 in]
            n90 = case shown="\"CONNECTION_RECONNECT\"" w193 {
              tunnel: [_ "UI: Cursor Set >> Busy\nConnections: Terminate\nConnections: Initialize\nUI: Cursor Set >> Idle" "UI: Connections Status" "Camera: Crop" "Camera: Auto Focus" "Tools: Sensor Readout" "UI: Help >> About" _ "UI: Cursor Set >> Busy\nUI: StatusString >> Checking for Updates\nCore: Check Update >> Display\nUI: StatusString >> Idle\nUI: Cursor Set >> Idle" "Data: Config" "Data: Open Folder" "Data: Calibration" "Macro: Exit" "Data: Options" "Data: Options Vision" "Data: Options PID" w230 _ "System: Override" "UI: Chart Clear\nUI: Chart Setup"] -> w192
              tunnel: w191 -> [w197 w198 w200 w202 w204 w206 w208 w210 w212 w214 w216 w218 w220 w222 w224 w226 w228 w240 w241 w243]
              tunnel: [w197 w198 w200 w202 w204 w206 w208 w210 w212 w214 w216 w218 w220 w222 w224 w226 w229 w240 w241 w243] -> w190
              frame "False", Default {
              }
              frame "CONNECTION_RECONNECT" {
              }
              frame "CONNECTION_STATUS" {
              }
              frame "CONTROL_CAMFEED" {
              }
              frame "CONTROL_CAMFOCUS" {
              }
              frame "CONTROL_DATA" {
              }
              frame "HELP_ABOUT" {
              }
              frame "HELP_MANUAL" {
                n91 = call-poly <vilib>:"Open URL in Default Browser.vi"("URL"="https://github.com/Aarhus-University-MPE/Ice-Nucleation-Controller/raw/main/docs/manual.pdf") -> ()  [unwired: 5 in, 2 out]
              }
              frame "HELP_UPDATE" {
              }
              frame "SETUP_CONFIG" {
              }
              frame "SETUP_FOLDER" {
              }
              frame "SYSTEM_CALIBRATION" {
              }
              frame "SYSTEM_EXIT" {
              }
              frame "SYSTEM_OPTIONS" {
              }
              frame "SYSTEM_OPTIONS_VISION" {
              }
              frame "SYSTEM_OPTIONS_PID" {
              }
              frame "SYSTEM_AUTOPID" {
                n92 = call "System_Ready.vi"("DataCluster"=w228) -> ("Data Acquisition Ready"=w231:bool)
                n93 = local write "Start"(w231) -> ()
                n94 = case shown="True" w231 {
                  tunnel: ["UI: Connections Status" ("State(s) in Front (\"\")") "System: Start\nUI: Autotune >> Diable\nSystem: Disable Autotune" ("State(s) in Front (\"\")")] -> w230
                  tunnel: w228 -> [w232 w236]
                  tunnel: [w232 w235] -> w229
                  frame False {
                  }
                  frame True {
                    n95 = Bundle By Name(cluster=w236, "Control.PID.AutoPID"=TRUE) -> (w235:T2)
                  }
                }
              }
              frame "SYSTEM_OVERHEAD" {
                n96 = property on="DP_Overhead" class="WFChart (strict)"() -> ("Visible"=w239:bool)  [unwired: 2 in, 2 out]
                n97 = Not(x=w239) -> (.not. x?=w238:bool)
                n98 = property on="DP_Overhead" class="WFChart (strict)"("Visible"=w238) -> ()  [unwired: 2 in, 2 out]
                n99 = property on="cDAQ_Time" class="WFChart (strict)"("Visible"=w238) -> ()  [unwired: 2 in, 2 out]
              }
              frame "SYSTEM_OVERRIDE" {
              }
              frame "UI_RESETGRAPH" {
              }
            }
            n100 = call <vilib>:"Add State(s) to Queue__JKI_lib_State_Machine.vi"("State(s) in Front (\"\")"=w192, "State(s) in (\"\")"=w196) -> ("States Out"=w195:string)  [unwired: 13 in]
          }
          event Panel Close? {
            # "Close Panel button (pressed) Event\n(this executes Macro: Exit to terminate the VI)"
            n101 = event-data() -> ()  [unwired: 1 in, 1 out]
            n102 = Bundle By Name(cluster=w249, "Core.Initialized?"=FALSE) -> (w246:T2)
            n103 = event-data("Discard?"=TRUE) -> ()  [unwired: 1 in, 1 out]
            n104 = call <vilib>:"Add State(s) to Queue__JKI_lib_State_Machine.vi"("State(s) in Front (\"\")"="Macro: Exit", "State(s) in (\"\")"=w252) -> ("States Out"=w251:string)  [unwired: 13 in]
          }
        }
      }
      frame "---------- Core ----------" {
        # "Do not put any code in this frame.\n(it is a separator no-op)"
        n105 = call <vilib>:"Add State(s) to Queue__JKI_lib_State_Machine.vi"("State(s) in (\"\")"=w256) -> ("States Out"=w255:string)  [unwired: 14 in]
      }
      frame Default {
        w266 = 42 items=["No error", "Argument error", "Memory is full", "Out of zone", "End of file", "File already open", "Generic file I/O error", "File not found", "File permission error", "Disk is full", "Duplicate path", "Too many files open", "System feature not enabled", "Resource file not found", "Cannot add resource", "Resource not found", "Image not found", "Image memory error", "Pen does not exist", "Config type invalid", "Config token not found", "Config parse error", "Config memory error", "Bad external code format", "Bad external code offset", "External code not present", "Null window", "Destroy window error", "Null menu", "Print aborted", "Bad print record", "Print driver error", "Windows error during printing", "Memory error during printing", "Print dialog error", "Generic print error", "Invalid device refnum", "Device not found", "Device parameter error", "Device unit error", "Cannot open device", "Device call aborted", "Generic error", "Cancelled by user", "Object ID too low", "Object ID too high", "Object not in heap", "Unknown heap", "Unknown object (invalid DefProc)", "Unknown object (DefProc not in table)", "Message out of range", "Invalid (null) method", "Unknown message", "Manager call not supported", "Bad address", "Network operation in progress", "Network operation timed out", "Connection is busy", "Network attribute not supported", "Network error", "Address in use", "System out of memory", "Connection aborted", "Connection refused", "Not connected", "Already connected", "Connection closed", "Initialization error (interapplication manager)", "Bad occurrence", "Wait on unbound occurrence handler", "Occurrence queue overflow", "Datalog type conflict", "Unused", "Unrecognized type (interapplication manager)", "Memory corrupt", "Failed to make temporary DLL", "Old CIN version", "Drag socket not found", "Failed to load drop-object", "Failed to register OLE object", "Failed to release OLE object", "Format specifier type mismatch", "Unknown format specifier", "Too few format specifiers", "Too many format specifiers", "Scan failed", "Newer CIN version", "Error converting to variant", "Runtime menu error", "Password tampered", "Variant attribute not found", "Incompatible variant data type", "Event data is not available", "Event Store is not present", "Occurrence is not found", "Event Queue is not created", "Event info is not available", "Refnum passed is NULL", "Error retrieving Class GUID", "Error retrieving CoClass GUID", "Error retrieving TypeLib GUID.", "Bad built application magic bytes.", "Specific driver is different from the specific driver associated with the Logical Name.", "There is no session opened to the class driver.", "Max Error", "MAX - Error with config objects", "MAX - Error loading configuration", "MAX - Group not supported"]
        # "Current State"
        # "Do not delete, rename, or modify this frame.\n(this is used to capture unhandled states and typos)"
        # "Handle mistyped state name (developer tool)"
        n106 = Format Into String(format string="Software Exception: Unhandled State \"%s\"." ("message"), error in=w262, w257) -> (resulting string=w265:string, error out=w264:errorcluster)  [unwired: 1 in]
        n107 = call <vilib>:"Error Cluster From Error Code.vi"("show call chain? (False)"=TRUE, "error in (no error)"=w264, "error message (\"\")"=w265, "error code (0)"=w266) -> ("error out"=w263:errorcluster)  [unwired: 5 in]
        n108 = call <vilib>:"Add State(s) to Queue__JKI_lib_State_Machine.vi"("State(s) in (\"\")"=w261) -> ("States Out"=w260:string)  [unwired: 14 in]
      }
      frame "Core: Check Update" {
        # "Checks for updates released on GitHub\n(Prompts user on startup if current version is lower than latest release on GitHub)"
        n109 = call "System_Update_Check.vi"("error in (no error)"=w268, "Arguments"=w271) -> ("error out"=→"error out 3":errorcluster, "String"=→"version":string, "States Out"=w272:string)  [unwired: 7 in]
        n110 = call <vilib>:"Add State(s) to Queue__JKI_lib_State_Machine.vi"("State(s) in Front (\"\")"=w272, "State(s) in (\"\")"=w275) -> ("States Out"=w274:string)  [unwired: 13 in]
      }
      frame "Core: Update" {
        # "Display Update Prompt\n(Shows a popup to the user asking if they want to update, then opens link to download page on GitHub)"
        n111 = call "Read Exe Version.vi"("Application name"=path "BioSIM.exe") -> ("FileVersion"=w281:string)  [unwired: 7 in, 3 out]
        n112 = Concatenate Strings("Current version: " ("message"), w281, "\nLateset version: " ("string"), w283, "\nUpdate to newest version?" ("string")) -> (w278:string)
        n113 = Two Button Dialog(message=w278, 1:"Ignore" ("F button name (\"Cancel\")"), 2:"Update" ("T button name (\"OK\")")) -> (T button?=w280:bool)
        n114 = case shown="True" w280 {
          frame False {
          }
          frame True {
            n115 = call-poly <vilib>:"Open URL in Default Browser.vi"("URL"="https://github.com/Aarhus-University-MPE/BioSIM/releases/latest") -> ()  [unwired: 5 in, 2 out]
          }
        }
        n116 = call <vilib>:"Add State(s) to Queue__JKI_lib_State_Machine.vi"("State(s) in (\"\")"=w289) -> ("States Out"=w288:string)  [unwired: 14 in]
      }
      frame "Error Handler" {
        # "Unhandled Error -- Display it"
        # "Handle any errors here.\nYou can also output any states to clean-up after errors occur"
        # "Clear error"
        n117 = call <vilib>:"General Error Handler.vi"("error in (no error)"=w292) -> ()  [unwired: 10 in, 5 out]
        n118 = call <vilib>:"Add State(s) to Queue__JKI_lib_State_Machine.vi"("State(s) in Front (\"\")"="/* Post Error States", "State(s) in (\"\")"=w296) -> ("States Out"=w295:string)  [unwired: 13 in]
      }
      frame "Exit" {
        # "Do not put any code in this frame.\n(No errors that occur here will be handled.)"
        n119 = Bundle By Name(cluster=w299, "Core.Exit"=TRUE) -> (w297:T2)
        n120 = call <vilib>:"Add State(s) to Queue__JKI_lib_State_Machine.vi"("State(s) in (\"\")"=w303) -> ("States Out"=w302:string)  [unwired: 14 in]
      }
      frame "---------- Macro ----------" {
        # "Do not put any code in this frame.\n(It is a separator no-op. You can make a copy of this frame to create a new Macro frame)"
        n121 = call <vilib>:"Add State(s) to Queue__JKI_lib_State_Machine.vi"("State(s) in (\"\")"=w307) -> ("States Out"=w306:string)  [unwired: 14 in]
      }
      frame "Macro: Initialize" {
        # "Initialization Macro\n(This is called once, when the VI starts)"
        n122 = Current VI's Path() -> (path=w310:path)
        n123 = Open VI Reference(vi path=w310) -> (vi reference=w311:refnum<vi>)  [unwired: 5 in, 1 out]
        n124 = invoke class="VI" method="FP.Open"(reference=w311, "State"=T8."Hidden") -> (reference out=w308:refnum<vi>)  [unwired: 3 in, 4 out]
        n125 = Close Reference(reference=w308) -> ()  [unwired: 1 in, 1 out]
        n126 = call <vilib>:"Add State(s) to Queue__JKI_lib_State_Machine.vi"("State(s) in Front (\"\")"="UI: StatusString >> Initializing...\nUI: Cursor Set >> Busy\nUI: Start Button >> Connecting\nUI: StatusString >> Initializing Data\nData: Initialize\nLoading UI: Progress\nUI: StatusString >> Initializing Core Data\nData: Initialize Core Data\nLoading UI: Progress\nUI: StatusString >> Checking for Updates\nCore: Check Update\nLoading UI: Progress\nUI: StatusString >> Loading Calibration files\nData: Load Calibration\nUI: StatusString >> Initializing User Interface\nUI: Initialize\nLoading UI: Progress\nUI: StatusString >> Initializing Connections\nConnections: Initialize\nLoading UI: Progress\nUI: StatusString >> Finishing Initialization\nLoading UI: Exit\nUI: Front Panel State >> Normal\nUI: Cursor Set >> Idle\nUI: StatusString >> Idle", "State(s) in (\"\")"=w316) -> ("States Out"=w315:string)  [unwired: 13 in]
      }
      frame "Macro: Exit" {
        # "Exit Macro\n(This is called once, when the VI exits)"
        n127 = Unbundle By Name(w318) -> ("Core.Close Panel on Exit?"=w326:bool)
        n128 = Bundle By Name(cluster=w318, "Data Acquisition.Ready"=FALSE) -> (w317:T2)
        n129 = Select(t="UI: Front Panel State >> Close", s=w326, f="") -> (s? t:f=w323:string)
        n130 = call <vilib>:"Add State(s) to Queue__JKI_lib_State_Machine.vi"("State(s) in Front (\"\")"="UI: StatusString >> Closing System... Terminating Data Acquisition\nSystem: Stop\nUI: StatusString >> Closing System... Terminating Connections\nConnections: Terminate\nUI: StatusString >> Closing System... Data Cleanup\nData: Terminate\nUI: StatusString >> Closing System" ("State(s) in Front (\"\")"), "State(s) in (\"\")"=w323, "State(s) at Back (\"\")"="Exit") -> ("States Out"=w322:string)  [unwired: 12 in]
        n131 = call <vilib>:"Add State(s) to Queue__JKI_lib_State_Machine.vi"("State(s) in Front (\"\")"=w322, "State(s) in (\"\")"=w329) -> ("States Out"=w328:string)  [unwired: 13 in]
      }
      frame "---------- System ----------" {
        # "Template Separator\n(You can make a copy of, or modify, this frame)"
        n132 = call <vilib>:"Add State(s) to Queue__JKI_lib_State_Machine.vi"("State(s) in (\"\")"=w333) -> ("States Out"=w332:string)  [unwired: 14 in]
      }
      frame "System: Start" {
        # "Start Data Collection\n(Starts data collection and PID controlled levitator)"
        n133 = Unbundle By Name(w334) -> ("Data Acquisition.Ready"=w336:bool, "Data Acquisition.Active"=w337:bool)
        n134 = Not(x=w337) -> (.not. x?=w335:bool)
        n135 = And(x=w336, y=w335) -> (x .and. y?=w338:bool)
        n136 = case shown="True" w338 {
          selector: w338 -> [w345 _]
          tunnel: [w344 "UI: Cursor Set >> Busy \nUI: StatusString >> Clearing Chart\nUI: Chart Setup\nUI: Chart Clear\n// ----------- Data Files Setup ----------- //\nUI: StatusString >> Configuring Setup file\nData: Setup File Config\nUI: StatusString >> Configuring Data file\nData: Data File Config\nUI: StatusString >> Configuring Image Folder\nData: Image Folder Setup\n// ----------- Data Acquisition Setup----------- //\nUI: StatusString >> Initializing Buffer\nData Acquisition: Buffer Initialize\nUI: StatusString >> Starting Data Acquisition\nData Acquisition: Start\nUI: StatusString >> System Active\nUI: Time Left >> show\nUI: System Input >> disable\nUI: Cursor Set >> Idle" ("State(s) in Front (\"\")")] -> w339
          tunnel: w336 -> [w343 _]
          frame False {
            # "Systems not connected and ready"
            n137 = local write "Start"(w345) -> ()
            n138 = case shown="False" w343 {
              tunnel: ["UI: Connections Status" ("State(s) in Front (\"\")") "" ("State(s) in Front (\"\")")] -> w344
              frame False {
              }
              frame True {
              }
            }
          }
          frame True {
            # "System Connected and Ready"
          }
        }
        n139 = call <vilib>:"Add State(s) to Queue__JKI_lib_State_Machine.vi"("State(s) in Front (\"\")"=w339, "State(s) in (\"\")"=w342) -> ("States Out"=w341:string)  [unwired: 13 in]
      }
      frame "System: Stop" {
        # "Stop Data Collection.\n(Stops system data collection and PID controlled levitator)"
        n140 = local write "Start"(FALSE ("Start")) -> ()
        n141 = call "DataAcquisition_Stop_Master.vi"("Arguments"=w353, "DataCluster in"=w352) -> ("State(s) at Back"=w349:string, "State(s) in Front"=w350:string, "DataCluster out"=w351:T2)  [unwired: 7 in]
        n142 = call <vilib>:"Add State(s) to Queue__JKI_lib_State_Machine.vi"("State(s) in Front (\"\")"=w350, "State(s) in (\"\")"=w357, "State(s) at Back (\"\")"=w349) -> ("States Out"=w356:string)  [unwired: 12 in]
      }
      frame "System: State" {
        # "Set System State.\n(Sets or unsets system ready state)"
        n143 = case shown="\"ON\", Default" w358 {
          tunnel: [TRUE ("Data Acquisition.Ready") FALSE ("Data Acquisition.Ready")] -> w360
          frame "ON", Default {
          }
          frame "OFF" {
          }
        }
        n144 = Bundle By Name(cluster=w361, "Data Acquisition.Ready"=w360) -> (w359:T2)
        n145 = call <vilib>:"Add State(s) to Queue__JKI_lib_State_Machine.vi"("State(s) in (\"\")"=w364) -> ("States Out"=w363:string)  [unwired: 14 in]
      }
      frame "System: Disable Autotune" {
        # "Set System State.\n(Sets or unsets system ready state)"
        n146 = Bundle By Name(cluster=w371, "Control.PID.AutoPID"=FALSE) -> (w370:T2)
        n147 = call "Stall Data Flow.vim"("value in"=w370, "milliseconds to wait"=u32 500) -> ("value out"=w368:T2)  [unwired: 1 out]
        n148 = call <vilib>:"Add State(s) to Queue__JKI_lib_State_Machine.vi"("State(s) in (\"\")"=w374) -> ("States Out"=w373:string)  [unwired: 14 in]
      }
      frame "System: Delay" {
        # "Halt System For x ms\n(Callable system delay for specified time. Usage: System: Delay >> 500, for a 500 ms delay)"
        n149 = Decimal String To Number(string=w376) -> (number=w375:i32)  [unwired: 2 in, 1 out]
        n150 = Wait (ms)(milliseconds to wait=w375) -> ()  [unwired: 1 out]
        n151 = call <vilib>:"Add State(s) to Queue__JKI_lib_State_Machine.vi"("State(s) in (\"\")"=w380) -> ("States Out"=w379:string)  [unwired: 14 in]
      }
      frame "System: Override" {
        # "Override System Connection Status.\n(Allows access to most system components even without connections)"
        n152 = call <vilib>:"Add State(s) to Queue__JKI_lib_State_Machine.vi"("State(s) in Front (\"\")"="UI: Start Button >> Default\nUI: RTM >> CDAQ_SHOW\nUI: RTM >> CAM_SHOW\nUI: DC Status >> Ready\nUI: AC Status >> Ready\nUI: Temperature Status >> Active\nUI: Humidity Status >> Active\nSystem: State >> ON" ("State(s) in Front (\"\")"), "State(s) in (\"\")"=w385) -> ("States Out"=w384:string)  [unwired: 13 in]
      }
      frame "---------- Data ----------" {
        # "Do not put any code in this frame.\n(It is a separator no-op. You can make a copy of this frame to create a new Data frame)"
        n153 = call <vilib>:"Add State(s) to Queue__JKI_lib_State_Machine.vi"("State(s) in (\"\")"=w389) -> ("States Out"=w388:string)  [unwired: 14 in]
      }
      frame "Data: Initialize" {
        # "Initialize the core data, here.\n(data names are defined by what you wire into the bundle function)"
        n154 = call "Settings_Load.vi"("error in"=w394, "DefaultValues"=w390) -> ("error out"=w392:errorcluster, "DataCluster out"=w391:T2)  [unwired: 8 in]
        n155 = call "Data_Initialize.vi"("DataCluster in"=w391) -> ("DataCluster out"=w395:T2)  [unwired: 10 in]
        n156 = call <vilib>:"Add State(s) to Queue__JKI_lib_State_Machine.vi"("State(s) in Front (\"\")"="Data: Load Placeholder Image" ("State(s) in Front (\"\")"), "State(s) in (\"\")"=w397) -> ("States Out"=w396:string)  [unwired: 13 in]
      }
      frame "Data: Terminate" {
        # "Cleanup any data and references, here.\n(this is called automatically, by the Macro: Exit)"
        n157 = Bundle By Name(cluster=w403, "Data Acquisition.Camera.Calibration"=T9 {"Top Left"={"X"=0.0, "Y"=0.0}, "Top Right"={"X"=0.0, "Y"=0.0}, "Bottom Left"={"X"=0.0, "Y"=0.0}, "Bottom Right"={"X"=0.0, "Y"=0.0}, "Fixpoint"={"X"=0.0, "Y"=0.0}, "Scan Area"=0.0, "Fixpoint Area"=0.0, "Well Pixels"=[], "Valid"=FALSE}) -> (w400:T2)
        n158 = Unbundle By Name(w403) -> ("Core.Current VI Reference"=w404:refnum<vi>)
        n159 = call "Settings_Save.vi"("error in"=w399, "DataCluster"=w400) -> ("error out"=w398:errorcluster)  [unwired: 8 in, 1 out]
        n160 = Close Reference(reference=w404, error in (no error)=w398) -> (error out=w402:errorcluster)
        n161 = call <vilib>:"Add State(s) to Queue__JKI_lib_State_Machine.vi"("State(s) in (\"\")"=w406) -> ("States Out"=w405:string)  [unwired: 14 in]
      }
      frame "Data: Initialize Core Data" {
        # "Do not delete, rename, or modify this frame.\n(this is used to determine panel behavior on exit)"
        # "originally closed?"
        # "exe?"
        # "If panel starts closed or is an EXE, then close it when we exit"
        n162 = property class="VI"() -> ("FP.State"=w409:T8)  [unwired: 2 in, 2 out]
        n163 = property class="App"() -> ("App.Kind"=w415:T10)  [unwired: 2 in, 2 out]
        n164 = control-ref of="Current VI Reference"() -> (w410:refnum<vi>)
        n165 = Equal?(x=w409, y=T8."Closed" ("Front Panel Window:State")) -> (x = y?=w407:bool)
        n166 = Equal?(x=w415, y=T10."Run Time System" ("Application:Kind")) -> (x = y?=w413:bool)
        n167 = Or(x=w407, y=w413) -> (x .or. y?=w411:bool)
        n168 = Bundle By Name(cluster=w412, "Core.Current VI Reference"=w410, "Core.Close Panel on Exit?"=w411) -> (w417:T2)
        n169 = call <vilib>:"Add State(s) to Queue__JKI_lib_State_Machine.vi"("State(s) in (\"\")"=w419) -> ("States Out"=w418:string)  [unwired: 14 in]
      }
      frame "Data: Load Placeholder Image" {
        w426 = T14 4 items=["Grayscale (U8)", "Grayscale (I16)", "Grayscale (SGL)", "Complex (CSG)", "RGB (U32)", "HSL (U32)", "RGB (U64)", "Grayscale (U16)"] ("Image Type")
        w428 = "\\Resources\\camera_placeholder.png"  # \Resources\camera_placeholder.png
        # "Load Placeholder Image.\n(Initialize memory and load placeholder image)"
        n170 = call <vilib>:"Application Directory.vi"() -> ("Application Directory"=w430:path)
        n171 = Path To String(path=w430) -> (string=w432:string)
        n172 = call "IMAQ Create"("Image Name"="placeholder_img", "Image Type"=w426, "error in (no error)"=w422) -> ("New Image"=w429:T4, "error out"=w421:errorcluster)  [unwired: 2 in]
        n173 = Concatenate Strings(w432, w428) -> (w431:string)
        n174 = String To Path(string=w431) -> (path=w433:path)
        n175 = call "IMAQ ReadFile 2"("Use File Path Image Type"=FALSE, "File Path"=w433, "error in (no error)"=w421, "Image"=w429) -> ("error out"=w420:errorcluster, "Image Out"=w423:T4)  [unwired: 3 in, 3 out]
        n176 = local write "Camera Feed"(w423) -> ()
        n177 = Bundle By Name(cluster=w424, "Connections.Camera.Placeholder"=w423) -> (w434:T2)
        n178 = call <vilib>:"Add State(s) to Queue__JKI_lib_State_Machine.vi"("State(s) in (\"\")"=w436) -> ("States Out"=w435:string)  [unwired: 14 in]
      }
      frame "Data: Config" {
        # "Access Data Setup here.\n(this is called automatically, by the Settings Event Run time menu, and during Data Acquisition Start)"
        n179 = call "Settings_Config.vi"("DataCluster in"=w441) -> ("Canceled"=w438:bool, "DataCluster out"=w440:T2)  [unwired: 9 in]
        n180 = case shown="\"Start\"" w439 {
          tunnel: w438 -> [_ w449]
          tunnel: ["" w446] -> w437
          frame "False", Default {
          }
          frame "Start" {
            n181 = Select(t="System: Stop", s=w449, f="System: Start") -> (s? t:f=w446:string)
          }
        }
        n182 = call <vilib>:"Add State(s) to Queue__JKI_lib_State_Machine.vi"("State(s) in Front (\"\")"=w437, "State(s) in (\"\")"=w444) -> ("States Out"=w443:string)  [unwired: 13 in]
      }
      frame "Data: Partition" {
        # "Legacy code from Ice Nucleation Controller"
        # "Access Additional Data Setup here.\n(this is called automatically, by the Settings Event Run time menu, and during Data Acquisition Start)"
        n183 = call "Partition_Setup.vi"("DataCluster in"=w454) -> ("Canceled?"=w451:bool, "DataCluster out"=w453:T2)  [unwired: 8 in, 1 out]
        n184 = case shown="\"Start\"" w452 {
          tunnel: w451 -> [_ w462]
          tunnel: ["" w459] -> w450
          frame "False", Default {
          }
          frame "Start" {
            n185 = Select(t="System: Stop", s=w462, f="System: Start") -> (s? t:f=w459:string)
          }
        }
        n186 = call <vilib>:"Add State(s) to Queue__JKI_lib_State_Machine.vi"("State(s) in Front (\"\")"=w450, "State(s) in (\"\")"=w457) -> ("States Out"=w456:string)  [unwired: 13 in]
      }
      frame "Data: Options" {
        # "Access System Options here.\n(this is called automatically, by the Settings Event Run time menu)"
        n187 = call "Options.vi"("DataCluster in"=w466) -> ("State"=w464:string, "DataCluster out"=w465:T2)  [unwired: 9 in]
        n188 = call <vilib>:"Add State(s) to Queue__JKI_lib_State_Machine.vi"("State(s) in Front (\"\")"=w464, "State(s) in (\"\")"=w468) -> ("States Out"=w467:string)  [unwired: 13 in]
      }
      frame "Data: Options Vision" {
        # "Access System Options here.\n(this is called automatically, by the Settings Event Run time menu)"
        n189 = call "Options_CV.vi"("DataCluster in"=w472) -> ("State"=w470:string, "DataCluster out"=w471:T2)  [unwired: 9 in]
        n190 = call <vilib>:"Add State(s) to Queue__JKI_lib_State_Machine.vi"("State(s) in Front (\"\")"=w470, "State(s) in (\"\")"=w474) -> ("States Out"=w473:string)  [unwired: 13 in]
      }
      frame "Data: Options PID" {
        # "Access System Options here.\n(this is called automatically, by the Settings Event Run time menu)"
        n191 = call "Options_PID.vi"("DataCluster in"=w478) -> ("State"=w475:string, "DataCluster out"=w477:T2)  [unwired: 9 in]
        n192 = call <vilib>:"Add State(s) to Queue__JKI_lib_State_Machine.vi"("State(s) in Front (\"\")"=w475, "State(s) in (\"\")"=w480) -> ("States Out"=w479:string)  [unwired: 13 in]
      }
      frame "Data: Calibration" {
        # "Access Calibartion Settings here.\n(this is called automatically, by the Settings Event Run time menu)"
        n193 = call "Thermistor_Callibration.vi"("DataCluster in"=w483) -> ("State Out"=w481:string, "DataCluster out"=w482:T2)  [unwired: 9 in]
        n194 = call <vilib>:"Add State(s) to Queue__JKI_lib_State_Machine.vi"("State(s) in Front (\"\")"=w481, "State(s) in (\"\")"=w486) -> ("States Out"=w485:string)  [unwired: 13 in]
      }
      frame "Data: Load Calibration" {
        # "Load Calibration Data.\n(this is called automatically on startup)"
        n195 = call "Thermistor_Callibration_Load.vi"("error in"=w489, "DataCluster"=w491) -> ("error out"=w488:errorcluster, "State"=w487:string, "DataCluster out"=w490:T2)  [unwired: 7 in]
        n196 = call <vilib>:"Add State(s) to Queue__JKI_lib_State_Machine.vi"("State(s) in Front (\"\")"=w487, "State(s) in (\"\")"=w493) -> ("States Out"=w492:string)  [unwired: 13 in]
      }
      frame "Data: Save Calibration" {
        # "Save Calibration Data.\n(this is called automatically, once calibration settings are changed)"
        n197 = call "Thermistor_Callibration_Save.vi"("error in"=w496, "DataCluster"=w494) -> ("error out"=w495:errorcluster)  [unwired: 9 in]
        n198 = call <vilib>:"Add State(s) to Queue__JKI_lib_State_Machine.vi"("State(s) in (\"\")"=w498) -> ("States Out"=w497:string)  [unwired: 14 in]
      }
      frame "Data: Setup File Config" {
        # "Configure Setup File.\n(this is called automatically during data acquisition Start)"
        n199 = call "SetupFile_Create.vi"("error in (no error)"=w501, "DataCluster"=w502) -> ("error out"=w500:errorcluster, "DataCluster out"=w499:T2)  [unwired: 8 in]
        n200 = call <vilib>:"Add State(s) to Queue__JKI_lib_State_Machine.vi"("State(s) in (\"\")"=w504) -> ("States Out"=w503:string)  [unwired: 14 in]
      }
      frame "Data: Data File Config" {
        # "Configure Output Data File.\n(this is called automatically during data acquisition Start)"
        n201 = call "DataFile_Create.vi"("error in (no error)"=w506, "DataCluster"=w507) -> ("error out"=w505:errorcluster)  [unwired: 9 in]
        n202 = call <vilib>:"Add State(s) to Queue__JKI_lib_State_Machine.vi"("State(s) in (\"\")"=w509) -> ("States Out"=w508:string)  [unwired: 14 in]
      }
      frame "Data: Files Unlock" {
        # "Unlock Output Files.\n(this is called automatically during data acquisition Stop)"
        n203 = Unbundle By Name(w514) -> ("Data Acquisition.Setup.Label"=w522:string)
        n204 = call <vilib>:"Application Directory.vi"() -> ("Application Directory"=w520:path)
        n205 = Path To String(path=w520) -> (string=w521:string)
        n206 = Concatenate Strings(w521, "\\Data\\", w522) -> (w511:string)
        n207 = Concatenate Strings(w511, "\\Setup.csv") -> (w524:string)
        n208 = Concatenate Strings(w511, "\\Data.csv") -> (w523:string)
        n209 = String To Path(string=w524) -> (path=w525:path)
        n210 = String To Path(string=w523) -> (path=w526:path)
        n211 = Set Permissions(7:i16 448 ("permissions"), 8:w510, 11:w526) -> (0:w513:errorcluster)  [unwired: 2 in, 1 out]
        n212 = Set Permissions(7:i16 448 ("permissions"), 8:w513, 11:w525) -> (0:w512:errorcluster)  [unwired: 2 in, 1 out]
        n213 = call <vilib>:"Add State(s) to Queue__JKI_lib_State_Machine.vi"("State(s) in (\"\")"=w528) -> ("States Out"=w527:string)  [unwired: 14 in]
      }
      frame "Data: Stamp times" {
        # "Timestamp Setup File.\n(this is called automatically during data acquisition Stop)"
        n214 = call "SetupFile_Stamp.vi"("error in (no error)"=w531, "DataCluster"=w530) -> ("error out"=w532:errorcluster, "DataCluster out"=w529:T2)  [unwired: 8 in]
        n215 = call <vilib>:"Add State(s) to Queue__JKI_lib_State_Machine.vi"("State(s) in (\"\")"=w534) -> ("States Out"=w533:string)  [unwired: 14 in]
      }
      frame "Data: Open Folder" {
        # "Open Current Data Folder.\n(this is called from the runtime menu or shortcut - Ctrl + E)"
        n216 = Unbundle By Name(w543) -> ("Data Acquisition.Setup.Label"=w547:string)
        n217 = call <vilib>:"Application Directory.vi"() -> ("Application Directory"=w545:path)
        n218 = Path To String(path=w545) -> (string=w546:string)
        n219 = Concatenate Strings(w546, "\\Data\\", w547) -> (w542:string)
        n220 = String To Path(string=w542) -> (path=w540:path)
        n221 = Format Into String(format string="cmd /c start \"\" \"%s\"", w540) -> (resulting string=w539:string)  [unwired: 2 in, 1 out]
        n222 = call <vilib>:"System Exec.vi"("run minimized? (F)"=TRUE, "wait until completion? (T)"=FALSE, "error in (no error)"=w537, "command line"=w539) -> ("error out"=w536:errorcluster)  [unwired: 4 in, 3 out]
        n223 = call <vilib>:"Add State(s) to Queue__JKI_lib_State_Machine.vi"("State(s) in (\"\")"=w549) -> ("States Out"=w548:string)  [unwired: 14 in]
      }
      frame "Data: Image Folder Setup" {
        # "Configure Image Folder.\n(this is called automatically during data acquisition Start)"
        n224 = Unbundle By Name(w553) -> ("Data Acquisition.Setup.Label"=w555:string)
        n225 = call <vilib>:"Application Directory.vi"() -> ("Application Directory"=w562:path)
        n226 = Path To String(path=w562) -> (string=w561:string)
        n227 = Concatenate Strings(w561, "\\Data\\", w555, "\\Images\\" ("string")) -> (w559:string)
        n228 = String To Path(string=w559) -> (path=w558:path)
        n229 = call <vilib>:"Check if File or Folder Exists.vi"("error in (no error)"=w552, "path"=w558) -> ("error out"=w554:errorcluster, "file or folder exists?"=w557:bool, "dup path"=w556:path)  [unwired: 7 in]
        n230 = case shown="False" w557 {
          tunnel: w556 -> [w567 _]
          tunnel: w554 -> [w566 w568]
          tunnel: [w565 w568] -> w551
          frame False {
            n231 = Create Folder(path (use dialog)=w567, error in=w566) -> (error out=w565:errorcluster)  [unwired: 1 in, 2 out]
          }
          frame True {
          }
        }
        n232 = call <vilib>:"Add State(s) to Queue__JKI_lib_State_Machine.vi"("State(s) in (\"\")"=w564) -> ("States Out"=w563:string)  [unwired: 14 in]
      }
      frame "Data: Save Snapshot" {
        (unwired) string[] ["Timestamp", "V_AC", "F_AC", "V_DC", "Temp", "Humidity", "Dewpoint", "Air Temp"]
        # "Do not put any code in this frame.\n(It is a separator no-op. You can make a copy of this frame to create a new Data frame)"
        n233 = call "Snapshot_file_and_folder.vi"("DataCluster"=w592, "error in (no error)"=w591) -> ("File path"=w590:path, "error out"=w587:errorcluster)  [unwired: 1 out]
        n234 = Format Date/Time String(time format string (%c)="%H:%M:%S.%3U") -> (date/time string=w584:string)  [unwired: 2 in]
        n235 = property on="AC_Voltage" class="DigNum (strict)"() -> ("Value"=w583:dbl[unit])  [unwired: 2 in, 2 out]
        n236 = property on="AC_Freq" class="DigNum (strict)"() -> ("Value"=w582:dbl[unit])  [unwired: 2 in, 2 out]
        n237 = property on="DC_Voltage" class="DigNum (strict)"() -> ("Value"=w581:dbl[unit])  [unwired: 2 in, 2 out]
        n238 = property on="Temp" class="DigNum (strict)"() -> ("Value"=w580:dbl[unit])  [unwired: 2 in, 2 out]
        n239 = property on="Humidity" class="DigNum (strict)"() -> ("Value"=w579:dbl)  [unwired: 2 in, 2 out]
        n240 = property on="Dewpoint" class="DigNum (strict)"() -> ("Value"=w578:dbl)  [unwired: 2 in, 2 out]
        n241 = property on="Air Temp." class="DigNum (strict)"() -> ("Value"=w577:dbl)  [unwired: 2 in, 2 out]
        n242 = Format Into String(w583) -> (resulting string=w576:string)  [unwired: 3 in, 1 out]
        n243 = Format Into String(w582) -> (resulting string=w575:string)  [unwired: 3 in, 1 out]
        n244 = Format Into String(w581) -> (resulting string=w574:string)  [unwired: 3 in, 1 out]
        n245 = Format Into String(w580) -> (resulting string=w573:string)  [unwired: 3 in, 1 out]
        n246 = Format Into String(w579) -> (resulting string=w572:string)  [unwired: 3 in, 1 out]
        n247 = Format Into String(w578) -> (resulting string=w571:string)  [unwired: 3 in, 1 out]
        n248 = Format Into String(w577) -> (resulting string=w570:string)  [unwired: 3 in, 1 out]
        n249 = Build Array(w584, w576, w575, w574, w573, w572, w571, w570) -> (w569:string[])
        n250 = call-poly <vilib>:"Write Delimited Spreadsheet.vi"("file path (dialog if empty)"=w590, "1D data"=w569, "append to file? (new file:F)"=TRUE, "error in (no error)"=w587, "delimiter (\\t)"=";" ("delimiter (\\t)")) -> ("error out"=w586:errorcluster)  [unwired: 9 in, 1 out]
        n251 = call <vilib>:"Add State(s) to Queue__JKI_lib_State_Machine.vi"("State(s) in (\"\")"=w594) -> ("States Out"=w593:string)  [unwired: 14 in]
      }
      frame "---------- Connections ----------" {
        # "System Connections.\n(Handles master functions for connecting and disconnecting systems)"
        n252 = call <vilib>:"Add State(s) to Queue__JKI_lib_State_Machine.vi"("State(s) in (\"\")"=w598) -> ("States Out"=w597:string)  [unwired: 14 in]
      }
      frame "Connections: Initialize" {
        # "Initialize the System Connections, here.\n(this is called automatically, by the Macro: Init)"
        n253 = call <vilib>:"Add State(s) to Queue__JKI_lib_State_Machine.vi"("State(s) in Front (\"\")"="UI: StatusString >> Scanning for cDAQ\ncDAQ: Scan\nLoading UI: Progress\nUI: StatusString >> Connecting cDAQ\ncDAQ: Connect\nLoading UI: Progress\nUI: StatusString >> Connecting Camera\nCamera: Connect\nLoading UI: Progress\nUI: StatusString >> Connecting Humidity\nHumidity: Connect\nLoading UI: Progress\nUI: StatusString >> Validating Connections\nConnections: Status\nLoading UI: Progress\n// ----------- Data Acquisition Setup----------- //\nUI: StatusString >> Initializing cDAQ\ncDAQ: AI Initialize\ncDAQ: AO Initialize\ncDAQ: DO Initialize\nLoading UI: Progress\nUI: StatusString >> Initializing Camera\nCamera: Initialize\nLoading UI: Progress\nUI: Chart Clear\nUI: Chart Setup\nUI: Cursor Set >> Idle\nUI: StatusString >> Idle" ("State(s) in Front (\"\")"), "State(s) in (\"\")"=w603) -> ("States Out"=w602:string)  [unwired: 13 in]
      }
      frame "Connections: Terminate" {
        # "Terminate connection to DAQs and Power Supply (Peltier)"
        # "Terminate the System Connections, here.\n(this is called automatically, by the Macro: Exit)"
        n254 = Bundle By Name(cluster=w609, "Data Acquisition.Ready"=FALSE) -> (w605:T2)
        n255 = call "Stall Data Flow.vim"("value in"="UI: Cursor Set >> Busy\nUI: StatusString >> Terminating cDAQ Connection\ncDAQ: Disconnect\nUI: StatusString >> Terminating Camera Connection\nCamera: Terminate\nUI: StatusString >> Idle\nUI: Cursor Set >> Idle" ("State(s) in Front (\"\")"), "milliseconds to wait"=u32 250) -> ("value out"=w607:string)  [unwired: 1 out]
        n256 = call <vilib>:"Add State(s) to Queue__JKI_lib_State_Machine.vi"("State(s) in Front (\"\")"=w607, "State(s) in (\"\")"=w612) -> ("States Out"=w611:string)  [unwired: 13 in]
      }
      frame "Connections: Status" {
        # "Checks Connection Status.\n(this is called automatically, by the Connections: Initialize)"
        n257 = Unbundle By Name(w616) -> ("Connections.cDAQ DO.Connected"=w618:bool, "Connections.cDAQ AO.Connected"=w614:bool, "Connections.Camera.Connected"=w613:bool)
        n258 = Compound Arithmetic op=AND(w618, w614, w613) -> (w619:bool)
        n259 = case shown="True" w619 {
          selector: w619 -> [w623 w627]
          tunnel: ["UI: Start Button >> Error\nUI: StatusString >> Connection Error!" "Loading UI: Description >> Connections Successful\nUI: Start Button >> Default\nUI: StatusString >> Idle\nUI: DC Status >> Ready\nUI: AC Status >> Ready\nUI: Temperature Status >> Active\nUI: Humidity Status >> Active"] -> w617
          tunnel: w616 -> [w625 w629]
          tunnel: [w624 w628] -> w615
          frame False {
            n260 = Bundle By Name(cluster=w625, "Data Acquisition.Ready"=w623) -> (w624:T2)
          }
          frame True {
            n261 = Bundle By Name(cluster=w629, "Data Acquisition.Ready"=w627) -> (w628:T2)
          }
        }
        n262 = call <vilib>:"Add State(s) to Queue__JKI_lib_State_Machine.vi"("State(s) in Front (\"\")"=w617, "State(s) in (\"\")"=w622) -> ("States Out"=w621:string)  [unwired: 13 in]
      }
      frame "---------- cDAQ ----------" {
        # "Do not put any code in this frame.\n(It is a separator no-op. You can make a copy of this frame to create a new Data frame)"
        n263 = call <vilib>:"Add State(s) to Queue__JKI_lib_State_Machine.vi"("State(s) in (\"\")"=w634) -> ("States Out"=w633:string)  [unwired: 14 in]
      }
      frame "cDAQ: Scan" {
        # "Scan for cDAQ IDs\n(this is called automatically, by the Connections: Initialize)"
        n264 = call "CDAQ_Scan.vi"("DataCluster"=w636) -> ("DataCluster out"=w635:T2)  [unwired: 10 in]
        n265 = call <vilib>:"Add State(s) to Queue__JKI_lib_State_Machine.vi"("State(s) in (\"\")"=w639) -> ("States Out"=w638:string)  [unwired: 14 in]
      }
      frame "cDAQ: Connect" {
        # "Connect cDAQ.\n(this is called automatically, by the Connections: Initialize"
        n266 = call "cDAQ_Connect.vi"("DataCluster in"=w642) -> ("State"=w641:string, "DataCluster out"=w643:T2)  [unwired: 9 in]
        n267 = call <vilib>:"Add State(s) to Queue__JKI_lib_State_Machine.vi"("State(s) in Front (\"\")"=w641, "State(s) in (\"\")"=w645) -> ("States Out"=w644:string)  [unwired: 13 in]
      }
      frame "cDAQ: Disconnect" {
        # "Terminate cDAQ Connections.\n(this is called automatically, by the Macro: Exit)"
        n268 = call "cDAQ_Terminate.vi"("input cluster"=w647) -> ("output cluster"=w646:T2)  [unwired: 10 in]
        n269 = call <vilib>:"Add State(s) to Queue__JKI_lib_State_Machine.vi"("State(s) in (\"\")"=w650) -> ("States Out"=w649:string)  [unwired: 14 in]
      }
      frame "cDAQ: AO Initialize" {
        # "Initialize cDAQ Analog Output.\n(this is called automatically, by the Connections: Initialize"
        n270 = call "cDAQ_AO_Initialize.vi"("DataCluster"=w652) -> ("DataCluster out"=w651:T2)  [unwired: 10 in]
        n271 = call <vilib>:"Add State(s) to Queue__JKI_lib_State_Machine.vi"("State(s) in (\"\")"=w655) -> ("States Out"=w654:string)  [unwired: 14 in]
      }
      frame "cDAQ: AO Command" {
        # "Set cDAQ Analog Output.\n(this is called whenever manually setting any analog outputs, DC Volt, AC Volt, AC Freq)"
        n272 = call "cDAQ_AO_Write.vi"("DataCluster"=w657) -> ("DataCluster out"=w656:T2)  [unwired: 10 in]
        n273 = call <vilib>:"Add State(s) to Queue__JKI_lib_State_Machine.vi"("State(s) in (\"\")"=w660) -> ("States Out"=w659:string)  [unwired: 14 in]
      }
      frame "cDAQ: AO Pulse" {
        # "Output DC Pulse.\n(this is called when DC output is on and Pulse button is pressed)"
        n274 = call "DC_Pulse.vi"("Arguments"=w664, "DataCluster in"=w663) -> ("State(s) in Front"=w662:string, "DataCluster out"=w661:T2)  [unwired: 8 in]
        n275 = call <vilib>:"Add State(s) to Queue__JKI_lib_State_Machine.vi"("State(s) in Front (\"\")"=w662, "State(s) in (\"\")"=w667) -> ("States Out"=w666:string)  [unwired: 13 in]
      }
      frame "cDAQ: AI Initialize" {
        # "Initialize cDAQ Analog Output.\n(this is called automatically, by the Connections: Initialize"
        n276 = Unbundle By Name(w670) -> ("Connections.cDAQ AI.Task"=w671:refnum<k21>, "Connections.cDAQ AI.Connected"=w672:bool)
        n277 = case shown="True" w672 {
          tunnel: w671 -> [_ w678]
          tunnel: [FALSE TRUE] -> w669
          frame False {
          }
          frame True {
            n278 = call <vilib>:"DAQmx Start Task.vi"("task/channels in"=w678) -> ()  [unwired: 13 in, 2 out]
          }
        }
        n279 = Bundle By Name(cluster=w670, "Connections.cDAQ AI.Active"=w669) -> (w668:T2)
        n280 = call <vilib>:"Add State(s) to Queue__JKI_lib_State_Machine.vi"("State(s) in (\"\")"=w675) -> ("States Out"=w674:string)  [unwired: 14 in]
      }
      frame "cDAQ: DO Initialize" {
        # "Initialize cDAQ Digital Output.\n(this is called automatically, by the Connections: Initialize"
        n281 = call "cDAQ_DO_Initialize.vi"("DataCluster"=w680) -> ("DataCluster out"=w679:T2)  [unwired: 10 in]
        n282 = call <vilib>:"Add State(s) to Queue__JKI_lib_State_Machine.vi"("State(s) in (\"\")"=w683) -> ("States Out"=w682:string)  [unwired: 14 in]
      }
      frame "cDAQ: DO Command" {
        # "Set cDAQ Digital Output.\n(this is called when manually changing AC PSU State)"
        n283 = call "cDAQ_DO_Write.vi"("DataCluster"=w684) -> ()  [unwired: 11 in]
        n284 = call <vilib>:"Add State(s) to Queue__JKI_lib_State_Machine.vi"("State(s) in (\"\")"=w687) -> ("States Out"=w686:string)  [unwired: 14 in]
      }
      frame "---------- Humidity ----------" {
        # "Do not put any code in this frame.\n(It is a separator no-op. You can make a copy of this frame to create a new Data frame)"
        n285 = call <vilib>:"Add State(s) to Queue__JKI_lib_State_Machine.vi"("State(s) in (\"\")"=w691) -> ("States Out"=w690:string)  [unwired: 14 in]
      }
      frame "Humidity: Connect" {
        # "Connect Humidity Sensor.\n(this is called automatically, by the Macro: Init)"
        n286 = call "Humidity_Connect.vi"("error in (no error)"=w695, "DataCluster"=w697) -> ("error out"=w694:errorcluster, "Enum"=w693:T15, "DataCluster 2"=w696:T2)  [unwired: 5 in, 2 out]
        n287 = case shown="\"Faild to connect\", Default" w693 {
          tunnel: ["Loading UI: Description >> Humidity Sensor Connection Failed!\nUI: Humidity Status >> Offline" ("State(s) in Front (\"\")") "UI: Humidity Status >> Online" ("State(s) in Front (\"\")") "Humidity: Connect" ("State(s) in Front (\"\")")] -> w692
          frame "Faild to connect", Default {
          }
          frame "Connected" {
          }
          frame "Port wrong baud rate" {
          }
        }
        n288 = call <vilib>:"Add State(s) to Queue__JKI_lib_State_Machine.vi"("State(s) in Front (\"\")"=w692, "State(s) in (\"\")"=w699) -> ("States Out"=w698:string)  [unwired: 13 in]
      }
      frame "Humidity: Reading" {
        # "Do not put any code in this frame.\n(It is a separator no-op. You can make a copy of this frame to create a new Data frame)"
        n289 = call "Humidity_Read.vi"("error in (no error)"=w709, "Whait for val"=FALSE, "DataCluster"=w710) -> ("error out"=w708:errorcluster, "RH"=w706:dbl, "AT"=w703:dbl, "DP"=w704:dbl, "DataCluster 2"=w707:T2)  [unwired: 2 in, 2 out]
        n290 = local write "Dewpoint"(w704) -> ()
        n291 = local write "Air Temp."(w703) -> ()
        n292 = local write "Humidity"(w706) -> ()
        n293 = call <vilib>:"Add State(s) to Queue__JKI_lib_State_Machine.vi"("State(s) in (\"\")"=w712) -> ("States Out"=w711:string)  [unwired: 14 in]
      }
      frame "Humidity: Disconnect" {
        # "Terminate Humidity Connection.\n(this is called automatically, by the Macro: Exit)"
        n294 = Unbundle By Name(w714) -> ("Connections.Humidity.Port"=w715:refnum<visa-resource-name>, "Connections.Humidity.Connected"=w718:bool)
        n295 = case shown="True" w718 {
          tunnel: w717 -> [w723 w730]
          tunnel: [w723 w729] -> w716
          tunnel: w715 -> [_ w728]
          tunnel: w714 -> [w722 w727]
          tunnel: [w722 w724] -> w713
          frame False {
          }
          frame True {
            n296 = VISA Clear(VISA resource name=w728, error in (no error)=w730) -> (VISA resource name out=w731:refnum<visa-resource-name>, error out=w732:errorcluster)
            n297 = VISA Close(VISA resource name=w731, error in (no error)=w732) -> (error out=w729:errorcluster)
            n298 = Bundle By Name(cluster=w727, "Connections.Humidity.Port"=refnum<visa-resource-name> refnum, "Connections.Humidity.Connected"=FALSE) -> (w724:T2)
          }
        }
        n299 = call <vilib>:"Add State(s) to Queue__JKI_lib_State_Machine.vi"("State(s) in Front (\"\")"="UI: Humidity Status >> Offline" ("State(s) in Front (\"\")"), "State(s) in (\"\")"=w721) -> ("States Out"=w720:string)  [unwired: 13 in]
      }
      frame "---------- Camera ----------" {
        # "Do not put any code in this frame.\n(It is a separator no-op. You can make a copy of this frame to create a new Data frame)"
        n300 = call <vilib>:"Add State(s) to Queue__JKI_lib_State_Machine.vi"("State(s) in (\"\")"=w736) -> ("States Out"=w735:string)  [unwired: 14 in]
      }
      frame "Camera: Connect" {
        # "Initialize Camera Connection Connection.\n(this is called automatically, by the Connections: Initialize"
        n301 = call "TCam_Scan.vi"("error in"=w741, "input cluster"=w740) -> ("error out"=w738:errorcluster, "State out"=w737:string, "output cluster"=w739:T2)  [unwired: 7 in]
        n302 = call <vilib>:"Add State(s) to Queue__JKI_lib_State_Machine.vi"("State(s) in Front (\"\")"=w737, "State(s) in (\"\")"=w743) -> ("States Out"=w742:string)  [unwired: 13 in]
      }
      frame "Camera: Initialize" {
        # "Initialize Camera.\n(this is called automatically, by the Connections: Initialize)"
        n303 = Unbundle By Name(w745) -> ("Connections.Camera.Connected"=w744:bool)
        n304 = case shown="True" w744 {
          tunnel: [w751 w756] -> w748
          tunnel: w747 -> [w752 w755]
          tunnel: [w752 w754] -> w746
          tunnel: w745 -> [w751 w757]
          frame False {
          }
          frame True {
            n305 = call "Camera_Config.vi"("error in (no error)"=w755, "crop?"=TRUE, "DataCluster in"=w757) -> ("error out"=w754:errorcluster, "DataCluster out"=w756:T2)  [unwired: 7 in]
          }
        }
        n306 = call <vilib>:"Add State(s) to Queue__JKI_lib_State_Machine.vi"("State(s) in (\"\")"=w750) -> ("States Out"=w749:string)  [unwired: 14 in]
      }
      frame "Camera: Terminate" {
        # "Terminate Camera Config.\n(This should be called if camera acquisition will be halted)"
        n307 = Unbundle By Name(w762) -> ("Data Acquisition.Camera.Image"=w759:T4, "Connections.Camera.Session"=w764:T3, "Connections.Camera.Connected"=w760:bool)
        n308 = case shown="True" w760 {
          tunnel: w764 -> [_ w774]
          tunnel: w763 -> [w767 w773]
          tunnel: w762 -> [w768 w781]
          tunnel: [w768 w779] -> w761
          tunnel: w759 -> [_ w778]
          tunnel: [w767 w777] -> w758
          frame False {
          }
          frame True {
            n309 = call <vilib>:"IMAQdx Stop Acquisition.vi"("error in"=w773, "Session In"=w774) -> ("error out"=w772:errorcluster, "Session Out"=w775:T3)  [unwired: 8 in]
            n310 = call <vilib>:"IMAQdx Unconfigure Acquisition.vi"("error in"=w772, "Session In"=w775) -> ("error out"=w770:errorcluster, "Session Out"=w771:T3)  [unwired: 8 in]
            n311 = call <vilib>:"IMAQdx Close Camera.vi"("error in"=w770, "Session In"=w771) -> ("error out"=w769:errorcluster)  [unwired: 9 in]
            n312 = call "IMAQ Dispose"("All Images? (No)"=TRUE, "Image"=w778, "error in (no error)"=w769) -> ("error out"=w777:errorcluster)  [unwired: 3 in]
            n313 = Bundle By Name(cluster=w781, "Connections.Camera.Active"=FALSE) -> (w779:T2)
          }
        }
        n314 = call <vilib>:"Add State(s) to Queue__JKI_lib_State_Machine.vi"("State(s) in (\"\")"=w766) -> ("States Out"=w765:string)  [unwired: 14 in]
      }
      frame "Camera: Disconnect" {
        # "Terminate Camera Connection.\n(this is called automatically, by the Macro: Exit)"
        n315 = Unbundle By Name(w785) -> ("Connections.Camera.Session"=w786:T3, "Connections.Camera.Connected"=w787:bool)
        n316 = case shown="True" w787 {
          tunnel: w786 -> [_ w794]
          tunnel: w785 -> [w791 w797]
          tunnel: [w791 w795] -> w784
          tunnel: w783 -> [w790 w793]
          tunnel: [w790 w792] -> w782
          frame False {
          }
          frame True {
            n317 = call <vilib>:"IMAQdx Close Camera.vi"("error in"=w793, "Session In"=w794) -> ("error out"=w792:errorcluster)  [unwired: 9 in]
            n318 = Bundle By Name(cluster=w797, "Connections.Camera.Connected"=FALSE ("Connections.cDAQ.Connected")) -> (w795:T2)
          }
        }
        n319 = call <vilib>:"Add State(s) to Queue__JKI_lib_State_Machine.vi"("State(s) in (\"\")"=w789) -> ("States Out"=w788:string)  [unwired: 14 in]
      }
      frame "Camera: Load Calibration" {
        # "Load Camera Calibration.\n(This is an unused function)"
        n320 = call "TCam_CalibrationLoad.vi"("error in (no error)"=w800, "DataCluster"=w802) -> ("error out"=w799:errorcluster, "state out"=w798:string, "output cluster"=w801:T2)  [unwired: 7 in]
        n321 = call <vilib>:"Add State(s) to Queue__JKI_lib_State_Machine.vi"("State(s) in Front (\"\")"=w798, "State(s) in (\"\")"=w804) -> ("States Out"=w803:string)  [unwired: 13 in]
      }
      frame "Camera: Auto Focus" {
        # "Unused with new camera"
        # "Run Camera Auto Focus.\n(This is called by the runtime menu function Auto Focus)"
        n322 = Unbundle By Name(w806) -> ("Connections.Camera.Session"=w810:T3, "Connections.Camera.Connected"=w809:bool)
        n323 = case shown="True" w809 {
          tunnel: w810 -> [_ w825]
          tunnel: w808 -> [w813 w824]
          tunnel: [w813 w821] -> w807
          tunnel: w806 -> [w814 w820]
          tunnel: [w814 w819] -> w805
          frame False {
          }
          frame True {
            n324 = property class="IMAQdx"(reference=w825, error in=w824, "ActiveAttribute"="AutoFocus", "ValueBool"=TRUE) -> (reference out=w817:T3, error out=w822:errorcluster)
            n325 = call "Stall Data Flow.vim"("value in"=w817, "milliseconds to wait"=u32 2000) -> ("value out"=w816:T3)  [unwired: 1 out]
            n326 = property class="IMAQdx"(reference=w816, error in=w822, "ActiveAttribute"="FocusPos") -> (error out=w821:errorcluster, "ValueU32"=w818:u32)  [unwired: 1 out]
            n327 = Bundle By Name(cluster=w820, "Data Acquisition.Camera.FocusPos"=w818) -> (w819:T2)
          }
        }
        n328 = call <vilib>:"Add State(s) to Queue__JKI_lib_State_Machine.vi"("State(s) in (\"\")"=w812) -> ("States Out"=w811:string)  [unwired: 14 in]
      }
      frame "Camera: Crop" {
        # "Open Camera Crop Window.\n(Opens separate window to configure camera crop, executed from runtime menu)"
        n329 = call "Camera_Feed.vi"("error in"=w831, "DataCluster"=w832) -> ("error out"=w830:errorcluster, "State(s) in Front"=w828:string, "DataCluster out"=w829:T2)  [unwired: 7 in]
        n330 = call <vilib>:"Add State(s) to Queue__JKI_lib_State_Machine.vi"("State(s) in Front (\"\")"=w828, "State(s) in (\"\")"=w834) -> ("States Out"=w833:string)  [unwired: 13 in]
      }
      frame "---------- Data Acquisition ----------" {
        # "Template Separator\n(You can make a copy of, or modify, this frame)"
        n331 = call <vilib>:"Add State(s) to Queue__JKI_lib_State_Machine.vi"("State(s) in (\"\")"=w838) -> ("States Out"=w837:string)  [unwired: 14 in]
      }
      frame "Data Acquisition: Start" {
        # "Start Data Acquisition.\n(this is called automatically, by Start Data Acquisition)"
        n332 = Unbundle By Name(w840) -> ("Data Acquisition.Ready"=w846:bool, "Data Acquisition.Active"=w845:bool, "Control.DC PSU.Voltage"=w839:dbl[unit])
        n333 = Not(x=w845) -> (.not. x?=w847:bool)
        n334 = And(x=w846, y=w847) -> (x .and. y?=w841:bool)
        n335 = case shown="True" w841 {
          selector: w841 -> [w853 _]
          tunnel: [w852 _] -> w843
          tunnel: w840 -> [w851 w860]
          tunnel: [w851 w858] -> w844
          tunnel: w846 -> [w850 _]
          tunnel: w839 -> [_ w856]
          frame False {
            n336 = local write "Start"(w853) -> ()
            n337 = case shown="False" w850 {
              tunnel: ["UI: Connections Status" ("State(s) in Front (\"\")") "" ("State(s) in Front (\"\")")] -> w852
              frame False {
              }
              frame True {
              }
            }
          }
          frame True {
            n338 = Tick Count (ms)() -> (millisecond timer value=w857:u32)
            n339 = Bundle By Name(cluster=w860, "Data Acquisition.Active"=TRUE ("System.Active"), "Control.LogStart ms"=w857, "Control.DC PSU.Voltage Set"=w856) -> (w858:T2)
          }
        }
        n340 = call <vilib>:"Add State(s) to Queue__JKI_lib_State_Machine.vi"("State(s) in Front (\"\")"=w843, "State(s) in (\"\")"=w849) -> ("States Out"=w848:string)  [unwired: 13 in]
      }
      frame "Data Acquisition: Buffer Initialize" {
        # "Initialize Data Acquisition Buffer\n(Initialize Data Acquisition Buffer, executed automatically from Start Data acquisition)"
        n341 = call "Buffer_Initialize.vi"("error in (no error)"=w863, "DataCluster in"=w864) -> ("error out"=w862:errorcluster, "DataCluster Out"=w861:T2)  [unwired: 8 in]
        n342 = call <vilib>:"Add State(s) to Queue__JKI_lib_State_Machine.vi"("State(s) in (\"\")"=w866) -> ("States Out"=w865:string)  [unwired: 14 in]
      }
      frame "Data Acquisition: Buffer Terminate" {
        # "Terminate Data Acquisition Buffer\n(Terminates Data Acquisition Buffer, executed automatically from Stop Data acquisition)"
        n343 = Unbundle By Name(w867) -> ("Data Acquisition.Queue.Queue"=w868:refnum<queue>)
        n344 = Release Queue(queue=w868, force destroy? (F)=FALSE, error in (no error)=w870) -> (error out=w869:errorcluster)  [unwired: 2 out]
        n345 = call <vilib>:"Add State(s) to Queue__JKI_lib_State_Machine.vi"("State(s) in (\"\")"=w873) -> ("States Out"=w872:string)  [unwired: 14 in]
      }
      frame "---------- UI ----------" {
        # "Do not put any code in this frame.\n(It is a separator no-op. You can make a copy of this frame to create a new UI frame)"
        n346 = call <vilib>:"Add State(s) to Queue__JKI_lib_State_Machine.vi"("State(s) in (\"\")"=w877) -> ("States Out"=w876:string)  [unwired: 14 in]
      }
      frame "UI: Initialize" {
        w879 = u32 0 ("AC_Freq_Slide")
        w878 = FALSE ("Visible")
        # "Initialize the User Interface, here.\n(this is called automatically, by the Macro: Init)"
        n347 = control-ref of="This VI"() -> (w885:refnum<vi>)
        n348 = property class="VI" props=["Clone Name"](reference=w885) -> ()  [unwired: 1 in, 3 out]
        n349 = local write "Start"(FALSE ("Start")) -> ()
        n350 = property on="DP_Overhead" class="WFChart (strict)"("Visible"=w878) -> ()  [unwired: 2 in, 2 out]
        n351 = property on="cDAQ_Time" class="WFChart (strict)"("Visible"=w878) -> ()  [unwired: 2 in, 2 out]
        n352 = property on="Overload" class="Bool (strict)"("Visible"=w878) -> ()  [unwired: 2 in, 2 out]
        n353 = property on="DP_Overhead" class="WFChart (strict)"("History Data"=u32[] []) -> ()  [unwired: 2 in, 2 out]
        n354 = local write "DC_Voltage"(dbl[unit] 0.0 ("DC_Voltage")) -> ()
        n355 = local write "DC_Voltage_Slide"(w879) -> ()
        n356 = local write "AC_Freq"(dbl[unit] 100.0 ("AC_Freq")) -> ()
        n357 = local write "AC_Voltage"(dbl[unit] 0.0 ("AC_Voltage")) -> ()
        n358 = local write "AC_Freq_Slide"(w879) -> ()
        n359 = local write "AC_Voltage_Slide"(w879) -> ()
        n360 = call <vilib>:"Add State(s) to Queue__JKI_lib_State_Machine.vi"("State(s) in Front (\"\")"="UI: StatusString >> Clearing Chart History\nUI: Chart Setup\nUI: Chart Clear\nUI: Image Setup\nUI: DC Status >> Error\nUI: AC Status >> Error\nUI: Time Left >> hide\nUI: PID Controls\nUI: Autotune >> Enable" ("State(s) in Front (\"\")"), "State(s) in (\"\")"=w892) -> ("States Out"=w891:string)  [unwired: 13 in]
        "Title" <- "BioSIM" ("Version")
        "Galium Control" <- "Galium Control" ("Galium Control")
      }
      frame "UI: StatusString" {
        # "Argument"
        # "Set Status String here\n(this is called takes argument and applies to Status String)"
        n361 = call <vilib>:"Add State(s) to Queue__JKI_lib_State_Machine.vi"("State(s) in (\"\")"=w897) -> ("States Out"=w896:string)  [unwired: 14 in]
        "StatusString" <- w893
      }
      frame "UI: Chart Setup" {
        # "Configure Chart\n(this is called automatically, by the Macro: Init)"
        n362 = property on="DC Volt" class="WFChart (strict)"("XScale.Maximum"=300.0 ("X Scale.Range:Maximum"), "XScale.Minimum"=0.0 ("X Scale.Range:Minimum"), "ActYScl"=0 ("Active Y Scale"), "YScale.Maximum"=1500.0 ("X Scale.Range:Maximum"), "YScale.Minimum"=0.0 ("X Scale.Range:Minimum")) -> ()  [unwired: 2 in, 2 out]
        n363 = property on="Temps" class="WFChart (strict)"("XScale.Maximum"=300.0 ("X Scale.Range:Maximum"), "XScale.Minimum"=0.0 ("X Scale.Range:Minimum"), "ActYScl"=0 ("Active Y Scale"), "YScale.Maximum"=30.0 ("Y Scale.Range:Maximum"), "YScale.Minimum"=-30.0 ("Y Scale.Range:Minimum")) -> ()  [unwired: 2 in, 2 out]
        n364 = call <vilib>:"Add State(s) to Queue__JKI_lib_State_Machine.vi"("State(s) in (\"\")"=w911) -> ("States Out"=w910:string)  [unwired: 14 in]
      }
      frame "UI: Chart Clear" {
        # "Clear Chart History.\n(this is called automatically, by the Macro: Init)"
        n365 = property on="DC Volt" class="WFChart (strict)"("History Data"=dbl[unit][] []) -> ()  [unwired: 2 in, 2 out]
        n366 = property on="Temps" class="WFChart (strict)"("History Data"=dbl[unit][] []) -> ()  [unwired: 2 in, 2 out]
        n367 = call <vilib>:"Add State(s) to Queue__JKI_lib_State_Machine.vi"("State(s) in (\"\")"=w917) -> ("States Out"=w916:string)  [unwired: 14 in]
      }
      frame "UI: Time Left" {
        # "Toggle Time Indicator\n(this is called automatically, by the Data Acquisition Start/Stop)"
        n368 = case shown="\"show\"" w919 {
          tunnel: [FALSE TRUE] -> w918
          frame "hide", Default {
          }
          frame "show" {
          }
        }
        n369 = property on="T_Log" class="Str"("Visible"=w918) -> ()  [unwired: 2 in, 2 out]
        n370 = call <vilib>:"Add State(s) to Queue__JKI_lib_State_Machine.vi"("State(s) in (\"\")"=w923) -> ("States Out"=w922:string)  [unwired: 14 in]
      }
      frame "UI: DC Status" {
        # "Configure DC Status Buttons\n(This shows/hides/configures DC PSU output buttons and labels)"
        n371 = case shown="\"Offline\", Default" w931 {
          selector: w931 -> [w939 w944 w949]
          tunnel: [u32 12333625 ("Text.Text Colors:Text Color") u32 3164499 ("Text.Text Colors:Text Color") u32 32768 ("Text.Text Colors:Text Color")] -> w930
          tunnel: [w939 w944 w949] -> w929
          tunnel: [T11."Disabled and Grayed Out" ("Disabled") T11."Enabled" ("Disabled") T11."Enabled" ("Disabled")] -> w927
          tunnel: [TRUE FALSE TRUE] -> w928
          tunnel: [FALSE FALSE TRUE] -> w926
          frame "Offline", Default {
          }
          frame "Ready" {
          }
          frame "Active" {
          }
        }
        "DC_Status" <- w929
        n372 = property on="DC_Voltage" class="DigNum (strict)"("DisabledEnum"=w927) -> ()  [unwired: 2 in, 2 out]
        n373 = property on="DC_Voltage_Slide" class="Slide (strict)"("DisabledEnum"=w927) -> ()  [unwired: 2 in, 2 out]
        n374 = property on="DC_Status" class="Str"("Text.TextColor"=w930, "Text.FontBold"=w928) -> ()  [unwired: 2 in, 2 out]
        n375 = property on="Pulse" class="Bool"("DisabledEnum"=w927, "Visible"=w926) -> ()  [unwired: 2 in, 2 out]
        n376 = call <vilib>:"Add State(s) to Queue__JKI_lib_State_Machine.vi"("State(s) in (\"\")"=w935) -> ("States Out"=w934:string)  [unwired: 14 in]
      }
      frame "UI: DC Update Values" {
        # "Update DC Values\n(Function called to update DC PSU Output Values)"
        n377 = Unbundle By Name(w953) -> ("Control.DC PSU.Voltage"=w951:dbl[unit])
        n378 = call "Convert_DC_VoltPct.vi"("DC_Volt"=w951) -> ("DC_Volt%"=w952:dbl)
        n379 = local write "DC_Voltage"(w951) -> ()
        n380 = local write "DC_Voltage_Slide"(w952) -> ()
        n381 = call <vilib>:"Add State(s) to Queue__JKI_lib_State_Machine.vi"("State(s) in (\"\")"=w956) -> ("States Out"=w955:string)  [unwired: 14 in]
      }
      frame "UI: System Input" {
        # "Argument"
        # "Toggles DC Voltage Input Buttons\n(This is called automatically by Data Acquisition Start/Stop, to enable/disable input during autonomy)"
        n382 = case shown="\"disable\"" w959 {
          tunnel: [w964 T11."Enabled" ("Disabled")] -> w958
          tunnel: [w964 T11."Disabled" ("Disabled")] -> w957
          frame "disable" {
            w964 = T11."Disabled" ("Disabled")
          }
          frame "enable", Default {
          }
        }
        n383 = property on="DC_Voltage" class="DigNum (strict)"("DisabledEnum"=w958) -> ()  [unwired: 2 in, 2 out]
        n384 = property on="DC_Voltage_Slide" class="Slide (strict)"("DisabledEnum"=w958) -> ()  [unwired: 2 in, 2 out]
        n385 = property on="Pulse" class="Bool"("DisabledEnum"=w958) -> ()  [unwired: 2 in, 2 out]
        n386 = property on="DC_Status" class="Str"("DisabledEnum"=w957) -> ()  [unwired: 2 in, 2 out]
        n387 = call <vilib>:"Add State(s) to Queue__JKI_lib_State_Machine.vi"("State(s) in (\"\")"=w963) -> ("States Out"=w962:string)  [unwired: 14 in]
      }
      frame "UI: PID Controls" {
        # "Toggles DC Voltage Input Buttons\n(This is called automatically by Data Acquisition Start/Stop, to enable/disable input during autonomy)"
        n388 = Unbundle By Name(w968) -> ("Control.PID.Show Controls"=w967:bool)
        n389 = property on="AutoTune" class="Bool"("Visible"=w967) -> ()  [unwired: 2 in, 2 out]
        n390 = property on="Auto Tune PID gains" class="Clust (strict)"("Visible"=w967) -> ()  [unwired: 2 in, 2 out]
        n391 = property on="TuneComplete" class="Bool (strict)"("Visible"=w967) -> ()  [unwired: 2 in, 2 out]
        n392 = call <vilib>:"Add State(s) to Queue__JKI_lib_State_Machine.vi"("State(s) in (\"\")"=w971) -> ("States Out"=w970:string)  [unwired: 14 in]
      }
      frame "UI: Autotune" {
        # "Toggles DC Voltage Input Buttons\n(This is called automatically by Data Acquisition Start/Stop, to enable/disable input during autonomy)"
        n393 = case shown="\"Disable\"" w972 {
          tunnel: [T11."Disabled and Grayed Out" ("Disabled") T11."Enabled" ("Disabled")] -> w973
          frame "Disable" {
          }
          frame "Enable", Default {
          }
        }
        n394 = property on="AutoTune" class="Bool"("DisabledEnum"=w973) -> ()  [unwired: 2 in, 2 out]
        n395 = call <vilib>:"Add State(s) to Queue__JKI_lib_State_Machine.vi"("State(s) in (\"\")"=w977) -> ("States Out"=w976:string)  [unwired: 14 in]
      }
      frame "UI: AC Status" {
        # "Configure AC Status Buttons\n(This shows/hides/configures AC PSU output buttons and labels)"
        n396 = case shown="\"Offline\", Default" w984 {
          selector: w984 -> [w991 w995 w999]
          tunnel: [u32 12333625 ("Text.Text Colors:Text Color") u32 3164499 ("Text.Text Colors:Text Color") u32 32768 ("Text.Text Colors:Text Color")] -> w982
          tunnel: [w991 w995 w999] -> w983
          tunnel: [T11."Disabled and Grayed Out" ("Disabled") T11."Enabled" ("Disabled") T11."Enabled" ("Disabled")] -> w980
          tunnel: [TRUE FALSE TRUE] -> w981
          frame "Offline", Default {
          }
          frame "Ready" {
          }
          frame "Active" {
          }
        }
        "AC_Status" <- w983
        n397 = property on="AC_Voltage" class="DigNum (strict)"("DisabledEnum"=w980) -> ()  [unwired: 2 in, 2 out]
        n398 = property on="AC_Voltage_Slide" class="Slide (strict)"("DisabledEnum"=w980) -> ()  [unwired: 2 in, 2 out]
        n399 = property on="AC_Freq" class="DigNum (strict)"("DisabledEnum"=w980) -> ()  [unwired: 2 in, 2 out]
        n400 = property on="AC_Freq_Slide" class="Slide (strict)"("DisabledEnum"=w980) -> ()  [unwired: 2 in, 2 out]
        n401 = property on="AC_Status" class="Str"("Text.TextColor"=w982, "Text.FontBold"=w981) -> ()  [unwired: 2 in, 2 out]
        n402 = call <vilib>:"Add State(s) to Queue__JKI_lib_State_Machine.vi"("State(s) in (\"\")"=w988) -> ("States Out"=w987:string)  [unwired: 14 in]
      }
      frame "UI: Temperature Status" {
        # "Configure Temp Status Buttons\n(This shows/hides/configures Temp buttons and labels)"
        n403 = case shown="\"Active\"" w1005 {
          selector: w1005 -> [w1012 _]
          tunnel: [u32 12333625 ("Text.Text Colors:Text Color") u32 32768 ("Text.Text Colors:Text Color")] -> w1003
          tunnel: [w1012 ""] -> w1004
          tunnel: [T11."Disabled and Grayed Out" ("Disabled") T11."Enabled" ("Disabled")] -> w1001
          tunnel: [TRUE TRUE] -> w1002
          frame "Offline", Default {
          }
          frame "Active" {
          }
        }
        "Temp Status" <- w1004
        n404 = property on="Temp" class="DigNum (strict)"("DisabledEnum"=w1001) -> ()  [unwired: 2 in, 2 out]
        n405 = property on="DC Volt" class="WFChart (strict)"("DisabledEnum"=w1001) -> ()  [unwired: 2 in, 2 out]
        n406 = property on="Temp Status" class="Str"("Text.TextColor"=w1003, "Text.FontBold"=w1002) -> ()  [unwired: 2 in, 2 out]
        n407 = call <vilib>:"Add State(s) to Queue__JKI_lib_State_Machine.vi"("State(s) in (\"\")"=w1009) -> ("States Out"=w1008:string)  [unwired: 14 in]
      }
      frame "UI: Humidity Status" {
        # "Configure Humidity Status Buttons\n(This shows/hides/configures Humidity buttons and labels)"
        n408 = case shown="\"Active\"" w1022 {
          selector: w1022 -> [w1029 _]
          tunnel: [u32 12333625 ("Text.Text Colors:Text Color") u32 32768 ("Text.Text Colors:Text Color")] -> w1020
          tunnel: [w1029 ""] -> w1021
          tunnel: [T11."Disabled and Grayed Out" ("Disabled") T11."Enabled" ("Disabled")] -> w1018
          tunnel: [TRUE TRUE] -> w1019
          frame "Offline", Default {
          }
          frame "Active" {
          }
        }
        "Humidity Status" <- w1021
        n409 = property on="Humidity" class="DigNum (strict)"("DisabledEnum"=w1018) -> ()  [unwired: 2 in, 2 out]
        n410 = property on="Temps" class="WFChart (strict)"("DisabledEnum"=w1018) -> ()  [unwired: 2 in, 2 out]
        n411 = property on="Humidity Status" class="Str"("Text.TextColor"=w1020, "Text.FontBold"=w1019) -> ()  [unwired: 2 in, 2 out]
        n412 = call <vilib>:"Add State(s) to Queue__JKI_lib_State_Machine.vi"("State(s) in (\"\")"=w1026) -> ("States Out"=w1025:string)  [unwired: 14 in]
      }
      frame "UI: Image Setup" {
        # "Configure Image Feed\n(Configures Display Mapping of Image feed)"
        n413 = Unbundle By Name(w1039) -> ("Data Acquisition.Camera.Display Mapping"=w1035:u32, "Control.Computer Vision.Display Image"=w1038:u32)
        n414 = case shown="0, Default" w1038 {
          tunnel: [TRUE FALSE] -> w1037
          frame 0, Default {
          }
          frame 1 {
          }
        }
        n415 = property on="Camera Feed" class="ImageControl"("16-bit Display Conversion Method"=w1035) -> ()  [unwired: 2 in, 2 out]
        n416 = Not(x=w1037) -> (.not. x?=w1036:bool)
        n417 = property on="Camera Feed" class="ImageControl"("Visible"=w1037) -> ()  [unwired: 2 in, 2 out]
        n418 = property on="Processing Feed" class="ImageControl"("Visible"=w1036) -> ()  [unwired: 2 in, 2 out]
        n419 = call <vilib>:"Add State(s) to Queue__JKI_lib_State_Machine.vi"("State(s) in (\"\")"=w1042) -> ("States Out"=w1041:string)  [unwired: 14 in]
      }
      frame "UI: Help" {
        # "Argument"
        # "UI Help Popup\n(This is called automatically when help button is pressed)"
        n420 = case shown="\"About\"" w1045 {
          frame "False", Default {
          }
          frame "About" {
            n421 = call "Read Exe Version.vi"("Application name"=path "BioSIM.exe") -> ("Build Date"=w1051:string, "FileVersion"=w1052:string)  [unwired: 7 in, 2 out]
            n422 = Concatenate Strings("Bioaerosol Simulation Chamber Control Software\n\nVersion: " ("message"), w1052, "\nBuilt on " ("message"), w1051) -> (w1054:string)
            n423 = One Button Dialog(message=w1054) -> ()  [unwired: 1 in, 1 out]
          }
        }
        n424 = call <vilib>:"Add State(s) to Queue__JKI_lib_State_Machine.vi"("State(s) in (\"\")"=w1049) -> ("States Out"=w1048:string)  [unwired: 14 in]
      }
      frame "UI: Popup" {
        # "Argument"
        # "Notification Popup\n(this is called takes argument and displays a popup)"
        n425 = One Button Dialog(message=w1056) -> ()  [unwired: 1 in, 1 out]
        n426 = call <vilib>:"Add State(s) to Queue__JKI_lib_State_Machine.vi"("State(s) in (\"\")"=w1060) -> ("States Out"=w1059:string)  [unwired: 14 in]
      }
      frame "UI: Alert" {
        # "Argument"
        # "UI Alert Popup\n(this function displays or pings different alerts to the user)"
        n427 = case shown="\"Done\"" w1061 {
          selector: w1061 -> [_ w1067]
          frame "Done" {
            n428 = call <vilib>:"Beep.vi"() -> ()  [unwired: 12 in]
            n429 = One Button Dialog(message="Target temperature reached") -> ()  [unwired: 1 in, 1 out]
          }
          frame Default {
            n430 = call <vilib>:"Beep.vi"() -> ()  [unwired: 12 in]
            n431 = One Button Dialog(message=w1067) -> ()  [unwired: 1 in, 1 out]
          }
        }
        n432 = call <vilib>:"Add State(s) to Queue__JKI_lib_State_Machine.vi"("State(s) in (\"\")"=w1065) -> ("States Out"=w1064:string)  [unwired: 14 in]
      }
      frame "UI: Connections Status" {
        # "Connection Status Popup\n(this function displays a connection status popup after pressing start button with connection errors)"
        n433 = call "ConnectionStatus.vi"("input cluster"=w1068) -> ("String"=w1069:string)  [unwired: 9 in, 1 out]
        n434 = call <vilib>:"Add State(s) to Queue__JKI_lib_State_Machine.vi"("State(s) in Front (\"\")"=w1069, "State(s) in (\"\")"=w1072) -> ("States Out"=w1071:string)  [unwired: 13 in]
      }
      frame "UI: Start Button" {
        # "Argument"
        # "Set Start Button Labels\n(this function toggles Start Button Labels and state based on connection status and data acquisition )"
        n435 = case shown="\"Error\"" w1075 {
          tunnel: [cluster{u32, u32}[] [{8388608, 8388608}, {4367360, 4367360}, {9342611, 9342611}, {6710891, 6710891}, {16711681, 16711680}, {16711681, 16711680}] ("Colors [4]") cluster{u32, u32}[] [{4367360, 12369084}, {10621999, 10621999}, {10621999, 10621999}, {4367360, 1985280}, {4367360, 1985280}, {10621999, 10621999}] ("Colors [4]") cluster{u32, u32}[] [{1985280, 12369084}, {4367360, 4367360}, {8388608, 16711681}, {1985280, 1985280}, {1985280, 4367360}, {8388608, 16711681}] ("Colors [4]")] -> _
          tunnel: [string[] ["Error", "Error", "Error", "Error"] ("Strings [4]") string[] ["Start", "Stop", "Stop", "Start"] ("Strings [4]") string[] ["Connecting", "Connecting", "Connecting", "Connecting"] ("Strings [4]")] -> w1074
          tunnel: [T11."Enabled" ("Disabled") T11."Enabled" ("Disabled") T11."Disabled" ("Disabled")] -> w1073
          frame "Error" {
          }
          frame "Default", Default {
          }
          frame "Connecting" {
          }
        }
        n436 = property on="Start" class="Bool (strict)"("Strings [4]"=w1074, "DisabledEnum"=w1073) -> ()  [unwired: 2 in, 2 out]
        n437 = call <vilib>:"Add State(s) to Queue__JKI_lib_State_Machine.vi"("State(s) in (\"\")"=w1079) -> ("States Out"=w1078:string)  [unwired: 14 in]
      }
      frame "UI: RTM" {
        # "Argument"
        # "Configure Runtime Menu\n(This function shows/hides different runtime menu buttons based on connection state of system)"
        n438 = Current VI's Menubar() -> (w1089:refnum<k9>)
        n439 = case shown="\"CAM_HIDE\"" w1090 {
          tunnel: w1089 -> [w1098 w1102 w1105 w1108 _ _]
          frame "CAM_SHOW" {
            w1095 = T11."Enabled" ("Disabled")
            n440 = Set Menu Item Info(7:"MENU_CAM" ("item name"), 9:TRUE ("enabled"), 11:w1098) -> ()  [unwired: 4 in, 2 out]
            n441 = property on="Camera Feed" class="ImageControl"("DisabledEnum"=w1095) -> ()  [unwired: 2 in, 2 out]
            n442 = property on="Processing Feed" class="ImageControl"("DisabledEnum"=w1095) -> ()  [unwired: 2 in, 2 out]
          }
          frame "CAM_HIDE" {
            w1099 = T11."Disabled and Grayed Out" ("Disabled")
            n443 = Set Menu Item Info(7:"MENU_CAM" ("item name"), 9:FALSE ("enabled"), 11:w1102) -> ()  [unwired: 4 in, 2 out]
            n444 = property on="Processing Feed" class="ImageControl"("DisabledEnum"=w1099) -> ()  [unwired: 2 in, 2 out]
            n445 = property on="Camera Feed" class="ImageControl"("DisabledEnum"=w1099) -> ()  [unwired: 2 in, 2 out]
          }
          frame "CDAQ_HIDE" {
            n446 = Set Menu Item Info(7:"MENU_CDAQ" ("item name"), 9:FALSE ("enabled"), 11:w1105) -> ()  [unwired: 4 in, 2 out]
          }
          frame "CDAQ_SHOW" {
            n447 = Set Menu Item Info(7:"MENU_CDAQ" ("item name"), 9:TRUE ("enabled"), 11:w1108) -> ()  [unwired: 4 in, 2 out]
          }
          frame "Default", Default {
          }
          frame "Connecting" {
          }
        }
        n448 = call <vilib>:"Add State(s) to Queue__JKI_lib_State_Machine.vi"("State(s) in (\"\")"=w1094) -> ("States Out"=w1093:string)  [unwired: 14 in]
      }
      frame "UI: Cursor Set" {
        # "Argument"
        # "Set and Unset Cursor Busy.\n(Usage: \"UI: Cursor Set >> Busy|Idle\")"
        n449 = case shown="\"Busy\"" w1109 {
          tunnel: w1111 -> [w1116 w1118]
          tunnel: [w1115 w1117] -> w1110
          frame "Idle", Default {
            n450 = call <vilib>:"Unset Busy.vi"("error in (no error)"=w1116) -> ("error out"=w1115:errorcluster)  [unwired: 10 in]
          }
          frame "Busy" {
            n451 = call <vilib>:"Set Busy.vi"("error in (no error)"=w1118) -> ("error out"=w1117:errorcluster)  [unwired: 9 in, 1 out]
          }
        }
        n452 = call <vilib>:"Add State(s) to Queue__JKI_lib_State_Machine.vi"("State(s) in (\"\")"=w1114) -> ("States Out"=w1113:string)  [unwired: 14 in]
      }
      frame "UI: Front Panel State" {
        # "Argument"
        # "Set Front Panel Open or Closed\n(Usage: \"UI: Front Panel State >> Open|Close\")"
        n453 = Unbundle By Name(w1121) -> ("Core.Current VI Reference"=w1120:refnum<vi>)
        n454 = case shown="\"Open\", \"Standard\", Default" w1119 {
          tunnel: w1123 -> [w1131 w1146 w1157 w1170 w1183]
          tunnel: [w1133 w1147 w1159 w1172 w1185] -> w1122
          tunnel: w1120 -> [w1132 w1144 w1158 w1171 w1184]
          frame "Open", "Standard", Default {
            w1126 = T8."Standard" ("State")
            n455 = property class="VI"(reference=w1132, error in=w1131) -> (reference out=w1129:refnum<vi>, error out=w1130:errorcluster, "FP.State"=w1128:T8)
            n456 = Not Equal?(x=w1128, y=w1126) -> (x != y?=w1127:bool)
            n457 = case shown="True" w1127 {
              tunnel: [w1137 w1139] -> w1133
              tunnel: w1130 -> [w1136 w1139]
              tunnel: w1129 -> [w1135 _]
              tunnel: w1126 -> [w1134 _]
              frame True {
                n458 = invoke class="VI" method="FP.Open"(reference=w1135, error in=w1136, "Activate"=TRUE, "State"=w1134) -> (error out=w1137:errorcluster)  [unwired: 1 in, 4 out]
              }
              frame False {
              }
            }
          }
          frame "Close", "Closed" {
            n459 = property class="VI"(reference=w1144, error in=w1146) -> (reference out=w1143:refnum<vi>, error out=w1145:errorcluster, "FP.State"=w1141:T8)
            n460 = Not Equal?(x=w1141, y=T8."Closed" ("Front Panel Window:State")) -> (x != y?=w1140:bool)
            n461 = case shown="True" w1140 {
              tunnel: [w1148 w1151] -> w1147
              tunnel: w1145 -> [w1148 w1150]
              tunnel: w1143 -> [_ w1149]
              frame False {
              }
              frame True {
                n462 = invoke class="VI" method="FP.Close"(reference=w1149, error in=w1150) -> (error out=w1151:errorcluster)  [unwired: 1 in, 2 out]
              }
            }
          }
          frame "Hidden", "Hide" {
            w1152 = T8."Hidden" ("State")
            n463 = property class="VI"(reference=w1158, error in=w1157) -> (reference out=w1155:refnum<vi>, error out=w1156:errorcluster, "FP.State"=w1154:T8)
            n464 = Not Equal?(x=w1154, y=w1152) -> (x != y?=w1153:bool)
            n465 = case shown="True" w1153 {
              tunnel: [w1163 w1164] -> w1159
              tunnel: w1156 -> [w1162 w1164]
              tunnel: w1155 -> [w1161 _]
              tunnel: w1152 -> [w1160 _]
              frame True {
                n466 = invoke class="VI" method="FP.Open"(reference=w1161, error in=w1162, "State"=w1160) -> (error out=w1163:errorcluster)  [unwired: 2 in, 4 out]
              }
              frame False {
              }
            }
          }
          frame "Minimize", "Minimized" {
            w1165 = T8."Minimized" ("State")
            n467 = property class="VI"(reference=w1171, error in=w1170) -> (reference out=w1168:refnum<vi>, error out=w1169:errorcluster, "FP.State"=w1167:T8)
            n468 = Not Equal?(x=w1167, y=w1165) -> (x != y?=w1166:bool)
            n469 = case shown="True" w1166 {
              tunnel: [w1176 w1177] -> w1172
              tunnel: w1169 -> [w1175 w1177]
              tunnel: w1168 -> [w1174 _]
              tunnel: w1165 -> [w1173 _]
              frame True {
                n470 = invoke class="VI" method="FP.Open"(reference=w1174, error in=w1175, "State"=w1173) -> (error out=w1176:errorcluster)  [unwired: 2 in, 4 out]
              }
              frame False {
              }
            }
          }
          frame "Maximize", "Maximized" {
            w1178 = T8."Maximized" ("State")
            n471 = property class="VI"(reference=w1184, error in=w1183) -> (reference out=w1181:refnum<vi>, error out=w1182:errorcluster, "FP.State"=w1180:T8)
            n472 = Not Equal?(x=w1180, y=w1178) -> (x != y?=w1179:bool)
            n473 = case shown="True" w1179 {
              tunnel: [w1189 w1190] -> w1185
              tunnel: w1182 -> [w1188 w1190]
              tunnel: w1181 -> [w1187 _]
              tunnel: w1178 -> [w1186 _]
              frame True {
                n474 = invoke class="VI" method="FP.Open"(reference=w1187, error in=w1188, "State"=w1186) -> (error out=w1189:errorcluster)  [unwired: 2 in, 4 out]
              }
              frame False {
              }
            }
          }
        }
        n475 = call <vilib>:"Add State(s) to Queue__JKI_lib_State_Machine.vi"("State(s) in (\"\")"=w1125) -> ("States Out"=w1124:string)  [unwired: 14 in]
      }
      frame "---------- Tools ----------" {
        # "Template Separator\n(You can make a copy of, or modify, this frame)"
        n476 = call <vilib>:"Add State(s) to Queue__JKI_lib_State_Machine.vi"("State(s) in (\"\")"=w1194) -> ("States Out"=w1193:string)  [unwired: 14 in]
      }
      frame "Tools: Sensor Readout" {
        # "Manual Sensor Readout.\n(Opens new window with manual sensor readouts)"
        n477 = call "Thermistor_Manual_Read.vi"("error in"=w1196, "input cluster"=w1197) -> ("error out"=w1195:errorcluster)  [unwired: 8 in, 1 out]
        n478 = call <vilib>:"Add State(s) to Queue__JKI_lib_State_Machine.vi"("State(s) in (\"\")"=w1199) -> ("States Out"=w1198:string)  [unwired: 14 in]
      }
      frame "Tools: PID" {
        # "PID Tuning.\n(Function to PID autonomous levitator)"
        n479 = call <vilib>:"Add State(s) to Queue__JKI_lib_State_Machine.vi"("State(s) in (\"\")"=w1203) -> ("States Out"=w1202:string)  [unwired: 14 in]
      }
      frame "Tools: Calibrate Thermal Camera" {
        # "Thermal Camera Calibration.\n(Opens Thermal Camera Calibration Software)"
        n480 = call <vilib>:"Application Directory.vi"() -> ("Application Directory"=w1208:path)
        n481 = Build Path(base path=w1208, name or relative path=path "TCC.exe") -> (appended path=w1206:path)
        n482 = Path To String(path=w1206) -> (string=w1205:string)
        n483 = call <vilib>:"System Exec.vi"("run minimized? (F)"=TRUE, "wait until completion? (T)"=FALSE, "command line"=w1205) -> ("error out"=→"error out":errorcluster)  [unwired: 5 in, 3 out]
        n484 = call <vilib>:"Add State(s) to Queue__JKI_lib_State_Machine.vi"("State(s) in (\"\")"=w1214) -> ("States Out"=w1213:string)  [unwired: 14 in]
      }
      frame "Tools: Temp Calc" {
        # "Thermal Camera Evaluation.\n(Opens Thermal Camera Evaluation Software)"
        n485 = call <vilib>:"Application Directory.vi"() -> ("Application Directory"=w1220:path)
        n486 = Build Path(base path=w1220, name or relative path=path "TCE.exe") -> (appended path=w1219:path)
        n487 = Path To String(path=w1219) -> (string=w1218:string)
        n488 = call <vilib>:"System Exec.vi"("run minimized? (F)"=TRUE, "wait until completion? (T)"=FALSE, "command line"=w1218) -> ("error out"=→"error out 2":errorcluster)  [unwired: 5 in, 3 out]
        n489 = call <vilib>:"Add State(s) to Queue__JKI_lib_State_Machine.vi"("State(s) in (\"\")"=w1225) -> ("States Out"=w1224:string)  [unwired: 14 in]
      }
      frame "---------- Loading UI ----------" {
        # "Do not put any code in this frame.\n(It is a separator no-op. You can make a copy of this frame to create a new UI frame)"
        n490 = call <vilib>:"Add State(s) to Queue__JKI_lib_State_Machine.vi"("State(s) in (\"\")"=w1229) -> ("States Out"=w1228:string)  [unwired: 14 in]
      }
      frame "Loading UI: Exit" {
        # "Loading Window Exit\n(This is the final state of the Loading Process, sets Initialized Flag to true)"
        n491 = Bundle By Name(cluster=w1232, "Core.Initialized?"=TRUE) -> (w1231:T2)
        n492 = call <vilib>:"Add State(s) to Queue__JKI_lib_State_Machine.vi"("State(s) in (\"\")"=w1235) -> ("States Out"=w1234:string)  [unwired: 14 in]
      }
      frame "Loading UI: Initialize" {
        # "Loading Window Initialize\n(This is the first state of the Loading Process, initializes Loading Window)"
        n493 = Bundle By Name(cluster=w1239, "Core.Initialized?"=FALSE) -> (w1238:T2)
        n494 = call <vilib>:"Add State(s) to Queue__JKI_lib_State_Machine.vi"("State(s) in Front (\"\")"="Loading Macro: Initialize" ("State(s) in Front (\"\")"), "State(s) in (\"\")"=w1242) -> ("States Out"=w1241:string)  [unwired: 13 in]
      }
      frame "Loading UI: Description" {
        # "Placeholder State\n(This state is not used, the state is run in the BioSim Loading Window)"
        n495 = call <vilib>:"Add State(s) to Queue__JKI_lib_State_Machine.vi"("State(s) in (\"\")"=w1246) -> ("States Out"=w1245:string)  [unwired: 14 in]
      }
      frame "Loading UI: Progress" {
        # "Placeholder State\n(This state is not used, the state is run in the BioSim Loading Window)"
        n496 = call <vilib>:"Add State(s) to Queue__JKI_lib_State_Machine.vi"("State(s) in (\"\")"=w1250) -> ("States Out"=w1249:string)  [unwired: 14 in]
      }
      frame "Loading UI: Version" {
        # "Placeholder State\n(This state is not used, the state is run in the BioSim Loading Window)"
        n497 = call <vilib>:"Add State(s) to Queue__JKI_lib_State_Machine.vi"("State(s) in (\"\")"=w1254) -> ("States Out"=w1253:string)  [unwired: 14 in]
      }
      frame "Loading Macro: Initialize" {
        # "Placeholder State\n(This state is not used, the state is run in the BioSim Loading Window)"
        n498 = call <vilib>:"Add State(s) to Queue__JKI_lib_State_Machine.vi"("State(s) in (\"\")"=w1258) -> ("States Out"=w1257:string)  [unwired: 14 in]
      }
    }
    n499 = call <extravilib>:"Write.vi"("element"=w10) -> ("channel"=w11:T16)  [unwired: 1 out]
  }
  n500 = call "LoadingWindow.vi"("channel"=w2) -> ()  [unwired: 11 in]
  n501 = while "Data Acquisition Loop" {
    tunnel: w1 -> [w1263]
    tunnel: w1 -> [w1262]
    stop <- w1259 stop-if-true
    n502 = call <extravilib>:"Read.vi"("channel"=w1263) -> ("element"=w1260:T2)  [unwired: 1 in, 1 out]
    n503 = call "System_Exit.vi"("DataCluster"=w1260) -> ("Exit"=w1259:bool)
    n504 = call "System_Ready.vi"("DataCluster"=w1260) -> ("Data Acquisition Ready"=w1261:bool)
    n505 = case shown="True" w1261 {
      tunnel: w1262 -> [_ w1269]
      tunnel: w1260 -> [_ w1266]
      frame False {
        # "System not Ready"
        n506 = Wait (ms)(milliseconds to wait=u32 100) -> ()  [unwired: 1 out]
      }
      frame True {
        # "System Ready"
        n507 = call "SampleRate_Convert.vi"("DataCluster"=w1266) -> ("Sample dt (ms)"=w1265:i64)  [unwired: 1 out]
        n508 = node-c288(w1265) -> (w1268:T17)  [unwired: 1 in]
        n509 = timed-loop {
          tunnel: w1269 -> [w1296]
          timing: w1268 -> [_]
          timing-out: [_] -> w1267
          stop <- w1287 stop-if-true
          n510 = node-c288() -> (w1294:i64)  [unwired: 1 in]
          n511 = call <extravilib>:"Read.vi"("channel"=w1296) -> ("element"=w1277:T2)  [unwired: 1 in, 1 out]
          n512 = call "System_Ready.vi"("DataCluster"=w1277) -> ("Data Acquisition Ready"=w1286:bool)
          n513 = call "timeleft_stamp.vi"("DataCluster"=w1277) -> ("Log Duration"=→"T_Log":string)
          n514 = call "System_Exit.vi"("DataCluster"=w1277) -> ("Exit"=w1276:bool)
          n515 = Not(x=w1286) -> (.not. x?=w1285:bool)
          n516 = Or(x=w1276, y=w1285) -> (x .or. y?=w1287:bool)
          n517 = call "CPU_Overload.vi"("Iteration Duration"=w1294, "DataCluster"=w1277) -> ("CPU_Overload?"=w1275:bool, "DP_Overhead"=→"DP_Overhead":i64)
          "Overload" <- w1275
          n518 = call "DAQ_Control.vi"("DataCluster"=w1277) -> ("DataCluster out"=w1278:T2, "AutoPID Cluster"=w1279:T20, "DAQ time"=→"cDAQ_Time":u32, "Sensor Cluster dup"=w1288:T21)  [unwired: 10 in, 1 out]
          n519 = Unbundle(w1279) -> ("tuning completed?"=→"TuneComplete":bool, "PID gains out"=→"Auto Tune PID gains":T1)
          n520 = call "SensorClusterUnpack.vi"("element"=w1278) -> ("Current Pos"=→"Position":dbl, "Processing"=→"Processing Feed":T4, "Image"=→"Camera Feed":T4, "DC Volt"=→"DC Volt":dbl[unit])  [unwired: 5 in]
          n521 = property on="Overload" class="Bool (strict)"("Visible"=w1275) -> ()  [unwired: 2 in, 2 out]
          n522 = Unbundle By Name(w1278) -> ("Control.DC PSU.Voltage"=w1280:dbl[unit])
          n523 = Unbundle By Name(w1288) -> ("Temp"=→"Temps" →"Temp":dbl[unit], "CMH"=w1273:T22)
          n524 = call "System_Active.vi"("DataCluster"=w1278) -> ("Data Acquisition Active"=w1281:bool)
          n525 = Unbundle By Name(w1273) -> ("Humidity"=→"Humidity":dbl, "Dewpoint"=→"Dewpoint":dbl, "Air Temp"=→"Air Temp.":dbl)
          n526 = case shown="True" w1281 {
            tunnel: w1280 -> [_ w1297]
            frame False {
            }
            frame True {
              n527 = call "Convert_DC_VoltPct.vi"("DC_Volt"=w1297) -> ("DC_Volt%"=w1298:dbl)
              n528 = local write "DC_Voltage"(w1297) -> ()
              n529 = local write "DC_Voltage_Slide"(w1298) -> ()
            }
          }
          n530 = node-c288() -> ()  [unwired: 1 out]
        }
        n531 = node-c288(w1267) -> ()
      }
    }
  }
  n532 = while "Data Logging Loop" {
    tunnel: w1 -> [w1310]
    tunnel: w1 -> [w1309]
    stop <- w1306 stop-if-true
    n533 = call <extravilib>:"Read.vi"("channel"=w1310) -> ("element"=w1307:T2)  [unwired: 1 in, 1 out]
    n534 = call "System_Exit.vi"("DataCluster"=w1307) -> ("Exit"=w1306:bool)
    n535 = call "System_Active.vi"("DataCluster"=w1307) -> ("Data Acquisition Active"=w1308:bool)
    n536 = case shown="True" w1308 {
      tunnel: w1309 -> [_ w1317]
      tunnel: w1307 -> [_ w1313]
      frame False {
        # "Data Acquisition Idle"
        n537 = Wait (ms)(milliseconds to wait=u32 100) -> ()  [unwired: 1 out]
      }
      frame True {
        # "Data Acquisition Active"
        n538 = node-c288(i64 50 ("Period")) -> (w1316:T17)  [unwired: 1 in]
        n539 = call "Camera_Frequency.vi"("DataCluster"=w1313) -> ("Image Frequency"=w1312:i32)
        n540 = timed-loop {
          tunnel: w1317 -> [w1322]
          shift-right: [w1319] -> _
          shift-left: w1312 -> [w1320]
          timing: w1316 -> [_]
          timing-out: [_] -> w1315
          stop <- w1321 stop-if-true
          # "Active Data Logging Loop"
          n541 = node-c288() -> ()  [unwired: 1 in]
          n542 = call <extravilib>:"Read.vi"("channel"=w1322) -> ("element"=w1318:T2)  [unwired: 1 in, 1 out]
          n543 = call "System_Inactive.vi"("DataCluster"=w1318) -> ("inactive/exit?"=w1321:bool)
          n544 = call "DataFile_Append.vi"("iteration"=w1320, "DataCluster"=w1318) -> ("iteration out"=w1319:i32)  [unwired: 9 in]
          n545 = node-c288() -> ()  [unwired: 1 out]
        }
        n546 = node-c288(w1315) -> ()  [unwired: 1 out]
      }
    }
  }
